vi "findmovablepath.vi"(8 "x":dbl) -> (0 "shift":dbl, 3 "theta handle":dbl=0.15)   [LabVIEW 2012]
uses:
  G_NAV.vi
  G_VEH.vi
  G_PATH.vi
  <vilib>/Analysis/Matrix/Numeric/Conversions/Array To Matrix - RA2.vi
  <vilib>/Analysis/7linalg.llb/Real SVD Decomposition.vi
  G_SEN.vi
  <vilib>/Analysis/NI_AALPro.lvlib
  <vilib>/Analysis/Matrix/NI_Matrix.lvlib
panel:
  out "M6006":T1={"GPSTime"=22892800.0, "attitude[2]"=-0.6123908, "lcc[0]"=-970.47205, "lcc[1]"=200.52362, "heading_GPS"=-0.6106907} {"GPSTime" format="%#_6f"}
  in  "Numeric":dbl
  out "sensor_obs":dbl[][](array[numeric])=[[-2.6493086559458767, 9.313377271515247, 0.316177936945349, -1.2], [-2.6066100840450477, 9.354542103994737, 0.3157590885476819, -1.2], [-2.579340659822815, 9.43207739327695, 0.31450254335468053, -1.2], [-2.6132527619437576, 9.439068677849818, 0.5859163050429868, 1.2000000000000006], [-2.6655003955140795, 9.41719146151926, 0.4953083793337705, 0.40000000000000013], [-2.8189313467074544, 9.344249551531279, 0.5859163050429868, 1.2000000000000006], [-2.5692189092921667, 9.480018973387281, 0.5863351534406539, 1.2000000000000006], [-2.6731933264342116, 9.434269134901442, 0.5863351534406539, 1.2000000000000006], [-2.77635346299322, 9.386711660550553, 0.5863351534406539, 1.2000000000000006], [-2.7290628288714722, 9.419794899689457, 0.5865445776394874, 1.2000000000000006], [-3.035140869949269, 9.26885391372332, 0.5865445776394874, 1.2000000000000006], [-2.550914688564252, 9.509578404068655, 0.3132459981616791, -1.2], [-2.785425991035746, 9.405948172518677, 0.495587629745689, 0.40000000000000013], [-2.7463409502228373, 9.457274042188466, 0.4957970675546278, 0.40000000000000013], [-2.90576588154835, 9.392310316924437, 0.49586688015760744, 0.40000000000000013], [-2.494747129058042, 9.597974241579312, 0.5880105470313224, 1.2000000000000006], [-2.836998990617639, 9.447892074399023, 0.4039934946364334, -0.3999999999999999], [-3.1184925197733824, 9.303796817000539, 0.5880105470313224, 1.2000000000000006], [-2.970577318209098, 9.393517402151646, 0.4960763179665463, 0.40000000000000013], [-2.9699981982750367, 9.392368449256733, 0.588219971230156, 1.2000000000000006], [-3.0729809459427746, 9.340776068194645, 0.4960763179665463, 0.40000000000000013], [-3.1996655181339673, 9.27234939560896, 0.40392368203345375, -0.3999999999999999], [-3.4973819131319495, 9.096981036828707, 0.40392368203345375, -0.3999999999999999], [-2.5289827185611418, 9.605504378157487, 0.3115706045710105, -1.2], [-3.453631348161608, 9.135814142218397, 0.4038538694304742, -0.3999999999999999], [-3.2339632015510937, 9.274656811335685, 0.5886388196278232, 1.2000000000000006], [-2.483097010676977, 9.64588076688389, 0.3111517561733434, -1.2], [-2.8803018639560647, 9.47148380231442, 0.4962857557754851, 0.40000000000000013], [-2.9317308980723027, 9.444962161904348, 0.5888482438266567, 1.2000000000000006], [-2.9582194094409178, 9.433270224287725, 0.4037142442245149, -0.3999999999999999], [-3.0350382771601945, 9.392890956174119, 0.5888482438266567, 1.2000000000000006], [-2.4599617564514022, 9.665942841266034, 0.5890576680254903, 1.2000000000000006], [-3.1930649800894275, 9.320188914278454, 0.5890576680254903, 1.2000000000000006], [-3.424919733239901, 9.200023640728578, 0.4035746190185557, -0.3999999999999999], [-3.4490855593711203, 9.183917089574846, 0.5892670922243238, 1.2000000000000006], [-2.6822275888719656, 9.595825896338217, 0.49649519358442396, 0.40000000000000013], [-3.1777999006997932, 9.352779338748892, 0.40350480641557607, -0.3999999999999999], [-3.3543988506422, 9.251882705008573, 0.5894765164231575, 1.2000000000000006], [-2.4169315260491846, 9.715129108585124, 0.589685940621991, 1.2000000000000006], [-2.4440270491484113, 9.70452412526726, 0.3103140593780091, -1.2], [-2.4445036099706936, 9.705733945395902, 0.40343499381259645, -0.3999999999999999], [-2.8187951120879293, 9.544925625371082, 0.40343499381259645, -0.3999999999999999], [-2.923864294836344, 9.494810195959495, 0.40343499381259645, -0.3999999999999999], [-3.4095769435307015, 9.230983589588824, 0.589685940621991, 1.2000000000000006], [-3.032582634559555, 9.45177853739907, 0.40336518120961684, -0.3999999999999999], [-3.2893092213922506, 9.313834366383366, 0.40336518120961684, -0.3999999999999999], [-3.313999270308597, 9.298296139668594, 0.5898953648208245, 1.2000000000000006], [-2.424651387634039, 9.734980699717582, 0.4967046313933628, 0.40000000000000013], [-2.533097518783729, 9.691715080471495, 0.4967046313933628, 0.40000000000000013], [-2.6407720438905313, 9.646563404831404, 0.4967046313933628, 0.40000000000000013], [-3.4004241638790518, 9.27277469308272, 0.4032255560036576, -0.3999999999999999], [-2.6217419806033297, 9.676437047583807, 0.403155743400678, -0.3999999999999999], [-2.6755410498513874, 9.653323143325384, 0.403155743400678, -0.3999999999999999], [-2.782523848427478, 9.605691332564723, 0.403155743400678, -0.3999999999999999], [-3.072259099823128, 9.465159649093863, 0.496844256599322, 0.40000000000000013], [-3.1500774192579093, 9.424433970288224, 0.403155743400678, -0.3999999999999999], [-3.605192513867668, 9.159018691750026, 0.403155743400678, -0.3999999999999999], [-2.5981277248582337, 9.69583138333276, 0.5907330616161588, 1.2000000000000006], [-3.102875064220138, 9.460567540591395, 0.4030859307976984, -0.3999999999999999], [-3.3599181191701257, 9.319548891673922, 0.4030859307976984, -0.3999999999999999], [-3.385278626883318, 9.304833131837459, 0.49691406920230163, 0.40000000000000013], [-2.5247869108477885, 9.749066890716904, 0.40294630559173916, -0.3999999999999999], [-2.5792234787521573, 9.726796302794572, 0.40294630559173916, -0.3999999999999999], [-3.551164984637863, 9.238618668727831, 0.5913613342126596, 1.2000000000000006], [-2.394482152160173, 9.820127604989409, 0.5915707584114931, 1.2000000000000006], [-2.7494727028492556, 9.675416799445248, 0.40280668038577994, -0.3999999999999999], [-3.681670154810481, 9.169274879714472, 0.40280668038577994, -0.3999999999999999], [-2.349619394154346, 9.868922054648976, 0.5921990310079939, 1.2000000000000006], [-2.625703441413957, 9.761592003343525, 0.497402757423159, 0.40000000000000013], [-3.2137622211581482, 9.48110235361721, 0.497402757423159, 0.40000000000000013], [-3.7275762623275384, 9.185498662423365, 0.5924084552068274, 1.2000000000000006], [-2.3569997188774257, 9.88892730018629, 0.4975423826291182, 0.40000000000000013], [-3.6331178758069624, 9.258143332791025, 0.5926178794056609, 1.2000000000000006], [-3.280263464375405, 9.479130763175284, 0.4976121952320978, 0.40000000000000013], [-2.450699178158054, 9.884289629873633, 0.30675384799783845, -1.2], [-2.4511770399787394, 9.885534502477135, 0.40224817956194303, -0.3999999999999999], [-2.5345511058394776, 9.852902522117958, 0.49775182043805705, 0.40000000000000013], [-3.824786250125524, 9.17047880734031, 0.40224817956194303, -0.3999999999999999], [-2.405397050205525, 9.933526651907876, 0.3061255754013377, -1.2], [-3.4089243051435196, 9.464380504252652, 0.4979612582469959, 0.40000000000000013], [-3.56907303823246, 9.381650335067114, 0.4980310708499755, 0.40000000000000013], [-3.532949127216187, 9.438353586460368, 0.49824050865891434, 0.40000000000000013], [-3.737313762681747, 9.3103050041449, 0.5947121213939967, 1.2000000000000006], [-2.2908474536598415, 10.059979664182297, 0.595549818189331, 1.2000000000000006], [-2.3765186719612967, 10.02943138812595, 0.3044501818106692, -1.2], [-2.462262709016492, 9.999031326649108, 0.4985197590708328, 0.40000000000000013], [-3.657097646318684, 9.409803942456133, 0.4985197590708328, 0.40000000000000013], [-3.835868568229564, 9.295365230962426, 0.40148024092916723, -0.3999999999999999], [-2.3581413988349413, 10.067967806625958, 0.5961780907858316, 1.2000000000000006], [-3.877029743260587, 9.302385055789298, 0.5961780907858316, 1.2000000000000006], [-3.9331436519651666, 9.276595165706414, 0.5963875149846652, 1.2000000000000006], [-3.425151432335213, 9.616047962173518, 0.4989386346887105, 0.40000000000000013], [-2.3143719287589564, 10.127343415537375, 0.49900844729169014, 0.40000000000000013], [-3.7975482431761254, 9.403949992407117, 0.49900844729169014, 0.40000000000000013], [-3.854407472044735, 9.378948406292697, 0.49907825989466975, 0.40000000000000013], [-2.407763132093687, 10.115274836822742, 0.4008519275023507, -0.3999999999999999], [-2.468901871015975, 10.10337801061548, 0.4007821148993711, -0.3999999999999999], [-2.3890129763037065, 10.15395227178771, 0.4993575103065882, 0.40000000000000013], [-3.777898705712374, 9.487607060347795, 0.4994273229095678, 0.40000000000000013], [-4.0346920104398265, 9.315984499311078, 0.5982723327741674, 1.2000000000000006], [-4.015722357091047, 9.342912286209264, 0.40050286448745265, -0.3999999999999999], [-2.372846250599384, 10.200711102617147, 0.30109939462933205, -1.2], [-2.3833228936159903, 10.23029622982958, 0.4001538014725545, -0.3999999999999999], [-3.9666747963375277, 9.4365483588187, 0.4998461985274455, 0.40000000000000013], [-2.30100181314674, 10.278532756817912, 0.5999477263648358, 1.2000000000000006], [-4.109576508398126, 9.423930057048132, 0.5003348867483028, 0.40000000000000013], [-2.35334151682133, 10.334600032038626, 0.2985863042433292, -1.2], [-4.074608378760497, 9.48436394539886, 0.5005443245572416, 0.40000000000000013], [-2.3368079650044735, 10.384014278769136, 0.5007537623661805, 0.40000000000000013], [-2.370078405901655, 10.38320748736416, 0.39917642503083994, -0.3999999999999999], [-4.204212822255533, 9.504238162023881, 0.3988273620159418, -0.3999999999999999], [-2.2707767805352264, 10.48873231405309, 0.2960732138573263, -1.2], [-2.3200348724405737, 10.53572713543776, 0.6051833313356751, 1.2000000000000006], [-2.245779677656643, 10.622703152908741, 0.29356012347132354, -1.2], [-2.279884830624796, 10.622358187824348, 0.6066493007275101, 1.2000000000000006], [-2.358065997017253, 10.651060149761754, 0.5025688900436505, 0.40000000000000013], [-2.206922249961846, 10.718517420078616, 0.29188472988065495, -1.2], [-2.310815072326706, 10.718984235455277, 0.5029179530585486, 0.40000000000000013], [-2.250256927274077, 10.7470116403635, 0.6089529669146794, 1.2000000000000006], [-2.4078141528407944, 10.696197951674801, 0.2910470330853207, -1.2], [-2.2625570787999116, 10.786624601979373, 0.5032670160734467, 0.40000000000000013], [-2.37319268235858, 10.803936049039782, 0.3963839209116553, -0.3999999999999999], [-2.4400133449020482, 10.792431192800741, 0.3963141083086757, -0.3999999999999999], [-2.3484550625403937, 10.948347869936686, 0.3954763570729203, -0.3999999999999999], [-2.2532005442925973, 10.986565753726355, 0.6137697234878515, 1.2000000000000006], [-2.2241527610867795, 11.130722431723722, 0.6164922380726879, 1.2000000000000006], [-2.3272220554510197, 11.112000353866012, 0.3944291680282261, -0.3999999999999999], [-2.2968682826047866, 11.131657762965752, 0.5056406445747536, 0.40000000000000013], [-2.2805508875817773, 11.32421563798276, 0.5068972714283867, 0.40000000000000013], [-2.3203488195890745, 11.3333663356091, 0.39296310336565415, -0.3999999999999999], [-2.2253235316083524, 11.390402063747686, 0.6217278430435271, 1.2000000000000006], [-2.23390046248441, 11.420813566670208, 0.5074557722522236, 0.40000000000000013], [-2.315297365324197, 11.574401473618405, 0.391357413497123, -0.3999999999999999], [-2.2168668356954866, 11.63137340411444, 0.6265445996166993, 1.2000000000000006], [-2.3994033185138965, 11.600249851280598, 0.2730365519856337, -1.2], [-2.233080590823236, 11.690844769333019, 0.5092708999296937, 0.40000000000000013], [-2.3589382981537037, 11.726595493110718, 0.27073288579846444, -1.2], [-2.3008663461775223, 11.796656013544418, 0.38989134883455107, -0.3999999999999999], [-2.209460232985442, 11.892117815907735, 0.6317802045875385, 1.2000000000000006], [-2.2516708194251622, 11.903349900014954, 0.3892630354077345, -0.3999999999999999], [-2.324463966690179, 11.881746284197003, 0.26780094701479445, -1.2], [-2.2175289279374653, 11.922764866099948, 0.5108067771952451, 0.40000000000000013], [-2.2538194745555633, 11.911368790129554, 0.2675915228159609, -1.2], [-2.178403555854863, 12.077484518563601, 0.5117841536369597, 0.40000000000000013], [-2.1829008579162608, 12.095192687788384, 0.6357592643653763, 1.2000000000000006], [-2.2383426880850124, 12.155028982889158, 0.3875875329362237, -0.3999999999999999], [-2.2804615843118747, 12.317890670472249, 0.25921455486261813, -1.2], [-2.2227746224162255, 12.415062075134333, 0.2575391612719496, -1.2], [-2.186230627716147, 12.434387153701119, 0.6426702629268841, 1.2000000000000006], [-2.196164124819029, 12.474982005763925, 0.5145068451531648, 0.40000000000000013], [-2.1425536546232067, 12.599100045840768, 0.6458116259093877, 1.2000000000000006], [-2.2643337612516414, 12.581746676789589, 0.3846554036110799, -0.3999999999999999], [-2.198573038349574, 12.65771577116447, 0.2527224046987775, -1.2], [-2.1750587039156537, 12.73714405461915, 0.5162521602276552, 0.40000000000000013], [-2.238686482838199, 12.824800292270476, 0.38304971374254876, -0.3999999999999999], [-2.1747996213790666, 12.920092091405744, 0.24748679972793824, -1.2], [-2.1535345564869504, 13.01725329936264, 0.6543980180615641, 1.2000000000000006], [-2.187058282696622, 13.165406851352257, 0.519184289552799, 0.40000000000000013], [-2.0682676188644926, 13.230434114169201, 0.24162292216059827, -1.2], [-2.249455724453499, 13.24346320074072, 0.3801873970203845, -0.3999999999999999], [-2.168249294443763, 13.280340530506738, 0.2401569527687633, -1.2], [-2.1361605605328022, 13.338559010168616, 0.6608901682254047, 1.2000000000000006], [-2.1577943406236098, 13.438198159944571, 0.520999417230269, 0.40000000000000013], [-2.1011219599138715, 13.601533356858653, 0.6661257731962439, 1.2000000000000006], [-2.2400954133839512, 13.604417430165359, 0.377743955916098, -0.3999999999999999], [-2.1622288912277443, 13.672487145254262, 0.3773948929011999, -0.3999999999999999], [-2.0809447496291567, 13.728170217410458, 0.23136113641775338, -1.2], [-2.148368119037393, 13.828678025980699, 0.5236522961434944, 0.40000000000000013], [-2.1431530665836362, 14.033933863880375, 0.37495145179691336, -0.3999999999999999], [-2.106513383233814, 14.090157922222986, 0.6761781347402553, 1.2000000000000006], [-2.116678410658171, 14.141260966031997, 0.5257466742328829, 0.40000000000000013], [-2.0736923856429295, 14.42245242291376, 0.6828797091029295, 1.2000000000000006], [-2.0946138788714483, 14.532649102029193, 0.5283995531461083, 0.40000000000000013], [-2.152273017194013, 14.572484794069997, 0.3712513838389937, -0.3999999999999999], [-2.0231688076393577, 14.688270075344283, 0.5293769295878229, 0.40000000000000013], [-2.0756120529212976, 14.699000478760663, 0.37048344520621795, -0.3999999999999999], [-2.0476810196035475, 14.823824383301131, 0.6910472528574387, 1.2000000000000006], [8.784462172926562, 11.47924364037722, 0.6985865240154472, 1.2000000000000006], [8.643867253715156, 11.631338367097312, 0.6985865240154472, 1.2000000000000006], [-2.01182307782236, 15.20812065601524, 0.5329373723397832, 0.40000000000000013], [8.86867671544905, 11.41559660678595, 0.6990053724131143, 1.2000000000000006], [8.58702381954077, 11.72028699299172, 0.6990053724131143, 1.2000000000000006], [8.952448256526495, 11.35108640713428, 0.6994242208107815, 1.2000000000000006], [8.751204607664915, 11.589530329880938, 0.699633645009615, 1.2000000000000006], [-2.0698358361213067, 15.238622346987988, 0.36678337724829835, -0.3999999999999999], [8.78228318958885, 11.618259075505645, 0.5334958731636202, 0.40000000000000013], [9.066064089233228, 11.311820599800757, 0.7006807660037829, 1.2000000000000006], [8.586576710391817, 11.864672700124274, 0.7010996144014501, 1.2000000000000006], [8.904607069385332, 11.588375580628155, 0.5339845613844775, 0.40000000000000013], [8.9823118978036, 11.517019884769494, 0.5340543739874571, 0.40000000000000013], [-2.038520846959818, 15.363492520347437, 0.7021467353956179, 1.2000000000000006], [8.791223365347536, 11.769957155305526, 0.5342638117963959, 0.40000000000000013], [8.577157812432615, 12.002632694506751, 0.7029844321909522, 1.2000000000000006], [9.089521761789143, 11.471296644949536, 0.5344034370023552, 0.40000000000000013], [8.747614402156172, 11.874019031613333, 0.5345430622083145, 0.40000000000000013], [9.196614789945517, 11.42431028033962, 0.5347525000172533, 0.40000000000000013], [8.702856524966558, 11.977947480441758, 0.5348223126202329, 0.40000000000000013], [8.551902917074258, 12.126859885849031, 0.7044504015827872, 1.2000000000000006], [9.301763328727434, 11.37452391977877, 0.7052880983781215, 1.2000000000000006], [8.546058430068586, 12.272774370500398, 0.7065446435711229, 1.2000000000000006], [8.713762205484503, 12.13805016075561, 0.5356600638559883, 0.40000000000000013], [9.379898466547676, 11.440670196564861, 0.5357996890619475, 0.40000000000000013], [8.680290014842434, 12.256372289618902, 0.536078939473866, 0.40000000000000013], [-1.9947666269032363, 15.748326418663561, 0.5366374402977029, 0.40000000000000013], [5.4033137061696035, 14.702228724352713, 0.7105237033489606, 1.2000000000000006], [5.31065139179097, 14.760192151279867, 0.5369166907096213, 0.40000000000000013], [5.318145573506214, 14.776082090179019, 0.7111519759454614, 1.2000000000000006], [5.372647557345696, 14.763989846509837, 0.36287387148143985, -0.3999999999999999], [5.430433378499369, 14.758453624273042, 0.5372657537245195, 0.40000000000000013], [5.282599535397169, 14.828571261939807, 0.3627342462754806, -0.3999999999999999], [-2.0630447970868317, 15.828269580660534, 0.3627342462754806, -0.3999999999999999], [-2.0425899368277762, 16.04197255374355, 0.7161781567174671, 1.2000000000000006], [8.986023479525567, 16.697743175440838, 0.7844504455372108, 1.2000000000000006], [8.870510744967275, 16.775657498704163, 0.7844504455372108, 1.2000000000000006], [8.776249405862337, 16.886004939029128, 0.7852881423325451, 1.2000000000000006], [9.255378545456706, 16.596057732863006, 0.7859164149290457, 1.2000000000000006], [9.146441633836046, 16.684541131912827, 0.7861258391278794, 1.2000000000000006], [9.094705994581439, 16.85736482840408, 0.5628171664150587, 0.40000000000000013], [9.445245140600367, 16.620273164434607, 0.7886389295138823, 1.2000000000000006], [8.745638718171325, 17.096618222434593, 0.7886389295138823, 1.2000000000000006], [9.250822015437112, 16.835004830220694, 0.563305854635916, 0.40000000000000013], [8.898582257650931, 17.072593546817984, 0.563305854635916, 0.40000000000000013], [9.372609476756939, 16.761935663932476, 0.5633756672388956, 0.40000000000000013], [9.022240713238299, 17.00273744358763, 0.5633756672388956, 0.40000000000000013], [9.671704217358442, 16.690540187776413, 0.79261798929172, 1.2000000000000006], [8.733353836557999, 17.341528099528503, 0.7928274134905535, 1.2000000000000006], [9.575618663038583, 16.801373411419853, 0.5644228562835899, 0.40000000000000013], [8.86635551362631, 17.284293500790973, 0.5644228562835899, 0.40000000000000013], [-11.730647795102412, 15.437193920648374, 0.09942389115260453, -1.2], [-11.753961919567294, 15.46091854606451, 0.3329242648031848, -0.3999999999999999], [-2.6376199176507695, 22.880864643377365, 0.586553451428128, 0.40000000000000013], [-2.8095170709695823, 22.87690194098971, 0.5866930766340872, 0.40000000000000013], [-2.472177558679492, 22.932903386537202, 0.5867628892370669, 0.40000000000000013], [-2.1457138125258957, 23.092372962417727, 0.5876006404728222, 0.40000000000000013], [-1.975660428365826, 23.120301035359756, 0.5876704530758019, 0.40000000000000013], [-2.830488522803034, 23.021539526550544, 0.8631939442986329, 1.2000000000000006], [-2.321307029798844, 23.112624067398425, 0.5878798908847407, 0.40000000000000013], [-2.664069979468923, 23.075216022238337, 0.8638222168951337, 1.2000000000000006], [-2.4981915740055283, 23.137390254704062, 0.864659913690468, 1.2000000000000006], [-2.3314305321547493, 23.198157106933053, 0.8654976104858023, 1.2000000000000006], [-1.8217528316749911, 23.325992950774253, 0.5889968925324145, 0.40000000000000013], [-2.1768599709453524, 23.37676650480826, 0.8688483976671393, 1.2000000000000006], [-15.001217509405912, 16.7719561296704, 0.31016535623183017, -0.3999999999999999], [-15.131558329077535, 16.65366297795977, 0.31002573102587094, -0.3999999999999999], [-14.921984448489132, 16.935815146369087, 0.30981629321693205, -0.3999999999999999], [-15.241790010790758, 16.749485916960253, 0.026963118356189475, -1.2], [-15.133075455565274, 16.88861418597005, 0.0267536941573559, -1.2], [-15.017973364486107, 17.261437164441947, 0.3077917277305232, -0.3999999999999999], [9.64601974480163, 21.452115753566822, 0.5922780848724565, 0.40000000000000013], [9.496453028675626, 21.54978831901161, 0.8772253656204823, 1.2000000000000006], [9.33857931433906, 21.631972172843444, 0.8772253656204823, 1.2000000000000006], [9.17999443103193, 21.712775206793534, 0.8772253656204823, 1.2000000000000006], [-15.156829567346312, 17.1472706411717, 0.022774634379518044, -1.2], [9.377029264437805, 21.70662736414938, 0.5929762109022526, 0.40000000000000013], [9.544865059367709, 21.641804454240944, 0.5931158361082118, 0.40000000000000013], [9.710389454590258, 21.571913609233842, 0.8797384560064849, 1.2000000000000006], [-1.8772014233671248, 23.929435618135358, 0.8797384560064849, 1.2000000000000006], [9.095883042737146, 21.944626194626313, 0.8807855770006529, 1.2000000000000006], [9.271801932592034, 21.894917952170292, 0.5938139621380081, 0.40000000000000013], [-15.236180272734178, 17.461386956855613, 0.017120181011011648, -1.2], [9.194957789557106, 22.145529906980062, 0.5951404015946207, 0.40000000000000013], [5.3379716006680615, 24.14040468850077, 0.30115953044745974, -0.3999999999999999], [5.346343602955266, 24.94301298686431, 0.29571414741504976, -0.3999999999999999], [-16.03827076279453, 20.400810973707614, 0.28733663505749585, -0.3999999999999999], [-15.917453817284267, 20.56937941691859, 0.2870573846455774, -0.3999999999999999], [-15.794914133758107, 20.737124067829413, 0.28677813423365894, -0.3999999999999999], [-14.857892347507073, 21.847969012040384, 0.2851724443651278, -0.3999999999999999], [-15.023801434595246, 21.725328510394597, 0.2851026317621482, -0.3999999999999999], [-15.339589077483758, 21.460351215716504, 0.2851026317621482, -0.3999999999999999], [-15.650704132941332, 21.189903024072276, 0.2851026317621482, -0.3999999999999999], [-15.201556508849778, 21.61650958244562, 0.28489319395320933, -0.3999999999999999], [-14.728337374906722, 22.016057756865447, 0.2848233813502297, -0.3999999999999999], [-15.626945243640977, 21.4767441096572, 0.28370637970255586, -0.3999999999999999], [9.50763508171292, 26.73975570562619, 0.6252994460818146, 0.40000000000000013], [-1.4252219468434035, 28.59895493907886, 0.6255088838907534, 0.40000000000000013], [9.725543674751258, 26.692789231824694, 0.6255786964937331, 0.40000000000000013], [9.943355423856874, 26.64378657215293, 0.6258579469056516, 0.40000000000000013], [9.334114379546264, 26.89614247546073, 0.6258579469056516, 0.40000000000000013], [9.216574706656742, 27.200382540182076, 0.6275334493771623, 0.40000000000000013], [10.040081267648652, 26.868922071117122, 0.9827751618326013, 1.2000000000000006], [-1.4946609322957394, 29.821814277404098, 1.0022516123241232, 1.2000000000000006], [9.883884675811041, 31.803099088007194, 0.6592981837328874, 0.40000000000000013], [9.665449175747526, 31.97349509801759, 0.659926497159704, 0.40000000000000013], [10.174424429491456, 31.838119222564067, 0.6602057475716224, 0.40000000000000013], [10.17244090528941, 31.83259465007272, 1.0805762626878783, 1.2000000000000006], [-1.0364518801246452, 37.42334336490329, 0.6869439745128152, 0.40000000000000013], [10.026103833352638, 36.8130958059697, 0.6928780457660825, 0.40000000000000013], [9.743408822772697, 36.92812129013003, 0.6930874835750214, 0.40000000000000013], [10.347031193921643, 36.82288619877287, 1.1808904539291583, 1.2000000000000006], [-21.069030510629236, 31.45954783569295, 0.20558607696836614, -0.3999999999999999], [-21.391355310423045, 31.377757000004777, 0.20467851312963112, -0.3999999999999999], [10.4210427571751, 41.72394225688742, 0.7265975330052368, 0.40000000000000013], [10.107451026305094, 41.89078819565647, 0.7271560338290737, 0.40000000000000013], [10.474235594988285, 41.919051326913184, 1.284136583954108, 1.2000000000000006], [10.13857155297352, 42.00899223589921, 1.284136583954108, 1.2000000000000006], [10.830210018606069, 41.90102810572798, 0.7285522858886659, 0.40000000000000013], [-0.709038750028526, 57.66347671663537, 1.5846603092802805, 1.2000000000000006], [11.120605021860856, 56.96437033164037, 0.8312466248716806, 0.40000000000000013], [-0.7151980727209852, 58.133987434462625, 0.8314560626806193, 0.40000000000000013], [1.5195348183779678, 61.52869356204023, 0.04473783970333195, -0.3999999999999999], [5.073212151726797, 61.48708023724171, 0.04362083805565814, -0.3999999999999999], [11.439817695944253, 61.011847285540675, 0.8593811038724656, 0.40000000000000013], [11.689176472740309, 65.06866600393317, 0.8875155828732506, 0.40000000000000013], [14.49832831315618, 65.07219891982305, 1.7750269060199955, 1.2000000000000006], [8.818111571073048, 72.81602044955893, 1.9136657256478184, 1.2000000000000006], [12.551831810983316, 72.91253923612891, 0.9424581014182081, 0.40000000000000013], [13.768405529858791, 72.71844886386302, 1.9283254195661683, 1.2000000000000006], [1.2476421313017925, 74.97736983119862, -0.04909029870127124, -0.3999999999999999], [0.9387629168292289, 75.21210795753403, 0.9506959885698028, 0.40000000000000013], [17.77975821366545, 76.1598746565128, 2.0169118556727685, 1.2000000000000006], [47.35648972259149, 63.571420836353425, 2.052304545275642, 1.2000000000000006], [13.031972557350265, 79.3416128979354, 2.061938058421986, 1.2000000000000006], [24.83184721270082, 81.07466865802802, 2.156178947897092, 1.2000000000000006], [13.551875448365177, 86.71163580640813, 1.0385900557211387, 0.40000000000000013], [52.872675769586, 69.37798867554798, 2.2194250559448303, 1.2000000000000006], [8.915518332671137, 92.0400907270114, 1.0712623539155988, 0.40000000000000013], [9.692181670683942, 91.99867908899289, 1.0715416043275172, 0.40000000000000013], [20.71894414488982, 95.06455786989261, 2.4164932270472192, 1.2000000000000006], [19.150342204408794, 95.56882049865551, 2.4198440142285564, 1.2000000000000006], [23.490178905085354, 95.9928006820069, 2.448953977866423, 1.2000000000000006], [26.036285319817722, 95.81770414584793, 2.4592157636092677, 1.2000000000000006], [14.717578948116746, 99.12164584891, 1.1254369338277803, 0.40000000000000013], [20.65463162219833, 155.2673630873944, 3.658378726130288, 1.2000000000000006], [12.312708261276875, 191.3556263648354, 4.393457664036117, 1.2000000000000006], [14.978259637770336, 232.0240814937235, 2.048848233439155, 0.40000000000000013], [33.73593705129936, 288.53349296533526, 2.4538311433239053, 0.40000000000000013], [8.92096999050232, 17.23708913161584, 0.3356469563193898, -0.3999999999999999], [-2.5256202703736608, 22.68399055587274, 0.31491261323444397, -0.3999999999999999], [-1.8996165215080512, 23.228271875851924, 0.3116314208944021, -0.3999999999999999], [-3.0296332585078587, 23.183843349397314, 0.8671730040764709, 1.2000000000000006], [5.104128617356655, 23.236200962780366, 0.022984058578351618, -1.2], [-1.2548826959515347, 24.01715071826592, 0.01942384719818102, -1.2], [5.221948215230284, 24.444090337557157, -0.0021468452816766903, -1.2], [-2.224688830349968, 25.593404278777417, 0.9151311456093583, 1.2000000000000006], [5.209357772395169, 25.198536731676327, -0.017434811796527283, -1.2], [-1.1725915542855405, 25.874379726198075, -0.019319629586029397, -1.2], [-15.005798944565672, 21.383214801932546, -0.039005504276384995, -1.2], [-14.976356804490646, 21.66777357175441, -0.04319398825305637, -1.2], [-14.955664951264778, 21.9687081224078, -0.04780132062739484, -1.2], [9.275033221452706, 26.45651279141699, 0.277143995022472, -0.3999999999999999], [9.363878146139614, 27.271589550954324, 0.2716287993870824, -0.3999999999999999], [9.371321144452127, 28.564736959442584, 0.26318147442654893, -0.3999999999999999], [10.747513637749273, 30.43885569655537, 1.0575396008161857, 1.2000000000000006], [11.012472531760006, 30.418068389611857, 1.0592149944068543, 1.2000000000000006], [11.266285997376329, 30.367042635463775, 1.060262115401022, 1.2000000000000006], [-20.735017036098906, 31.521767273772653, 0.20663326601306034, -0.3999999999999999], [-20.49557227262787, 31.709735125755284, 0.20656345341008076, -0.3999999999999999], [10.724864676049275, 37.00446773130826, 0.6956007372822874, 0.40000000000000013], [-21.806198041420327, 31.41066071306105, 0.20272376024620187, -0.3999999999999999], [10.97816933233072, 46.72664514439962, 0.7613642092890853, 0.40000000000000013], [-33.95444016665767, 37.454440166657676, 0.11475988049188635, -0.3999999999999999], [-33.46782468155926, 38.15694699438283, 0.11364287884421248, -0.3999999999999999], [-32.258000408687934, 39.32613895725404, 0.11343344103527364, -0.3999999999999999], [-34.39923085728631, 37.30403001674005, 0.11329381582931441, -0.3999999999999999], [11.618566184124763, 57.01187131155995, 0.8322938139163747, 0.40000000000000013], [16.615400312068406, 60.50485600252477, 1.6937703168725702, 1.2000000000000006], [13.205163345895427, 64.3192947748755, 1.7536656377389712, 1.2000000000000006], [20.538690765112868, 64.00503191176435, 1.7884300547453438, 1.2000000000000006], [13.026046392769018, 79.30712465157343, 0.9869985421192027, 0.40000000000000013], [27.29899080749756, 81.67230442986731, 2.1844512147396244, 1.2000000000000006], [33.69042505267091, 80.06731529671714, 2.2022522716404778, 1.2000000000000006], [29.157427120978678, 82.5346645544511, 2.2146082993716583, 1.2000000000000006], [27.17382907061827, 93.78874887901951, 2.425079619199396, 1.2000000000000006], [34.761055666251615, 92.88790635480824, 2.4590063394104344, 1.2000000000000006], [-2.729118001525531, 22.918683596868465, 0.31309748555697403, -0.3999999999999999], [9.124522914489708, 21.80096170236561, 0.3072332269066863, -0.3999999999999999], [-1.5170192378515415, 28.303045293335575, 0.2765156815956554, -0.3999999999999999], [-1.3900091234452605, 30.022954081648294, 0.2645777264861412, -0.3999999999999999], [4.034616118215339, 61.19769858054814, 0.04620390436590388, -0.3999999999999999], [26.121526235859253, 82.71602090547535, 2.197226090868472, 1.2000000000000006]]
  out "xplot":cluster{dbl[]}[](array[cluster])
  out "yplot":cluster{dbl[]}[](array[cluster])
  out "thetaseed":dbl[](array[numeric])
  out "center":i16
  out "right":i16
  out "left":i16
  out "XY Graph":cluster{"Y":dbl[], "Y":dbl[]}[](graph)=[{"Y"=[0.0], "Y"=[1000.0]}, {"Y"=[], "Y"=[]}, {"Y"=[], "Y"=[]}, {"Y"=[55.79381017995934], "Y"=[-143.41137512848826]}, {"Y"=[1.8243630881955273], "Y"=[-0.6091599202647308]}, {"Y"=[60.825233010671326, 56.37330625127248, 55.349089235151354, 59.801015994550255, 60.825233010671326], "Y"=[-144.72018116547483, -142.44414335187238, -144.44751039360185, -146.72354820720435, -144.72018116547483]}, {"Y"=[0.0, 2.210107140854234e-06, 8.840428449730098e-06, 1.9890964154001267e-05, 3.536171391260723e-05, 5.5252677611861145e-05, 7.956385525176302e-05, 0.00010829524660493917, 0.00014144685155770276, 0.0001790186695416196, 0.00022101070067037654, 0.00026742294460291305, 0.00031825540077079495, 0.00037350806894664856, 0.0004331809489031002, 0.0004972740399580289, 0.0005657873416566872, 0.0006387208537717015, 0.0007160745756209508, 0.0007978485066360008, 0.0008840426462484174, 0.0009746569938897665, 0.0010696915488779268, 0.0011691463105307776, 0.0012730212781661976, 0.001381316451102066, 0.0014940318285425747, 0.0016111674095782291, 0.0017327231935269083, 0.0018586991794791174, 0.001989095366525362, 0.00212391175364246, 0.002263148340148291, 0.0024068051247922995, 0.002554882106551304, 0.0027073792846294964, 0.002864296657776322, 0.003025634224741225, 0.003191391984614711, 0.0033615699362599116, 0.003536168078198898, 0.0037151864094084885, 0.003898624928524441, 0.004086483634296201, 0.004278762525359525, 0.004475461600350172, 0.0046765808579039, 0.004882120296656467, 0.0050920799150162566, 0.00530645971150534, 0.005525259684645789, 0.005748479832959674, 0.005976120154741693, 0.006208180648513917, 0.006444661312457356, 0.006685562145094082, 0.006930883144491418, 0.007180624309171435, 0.007434785636974084, 0.007693367126535122, 0.007956368775921874, 0.008223790583087975, 0.008495632546100751, 0.008771894663368585, 0.009052576932504053, 0.00933767935191554, 0.009627201919329309, 0.009921144632812684, 0.010219507490205615, 0.010522290489461739, 0.010829493628421005, 0.011141116904923365, 0.011457160316581394, 0.011777623861462416, 0.012102507536951634, 0.012431811341116372, 0.012765535271228146, 0.013103679325240591, 0.0134462435006526, 0.013793227794963059, 0.014144632205784546, 0.014500456730615952, 0.014860701366956164, 0.015225366112190386, 0.015594450963703821, 0.015967955919109045, 0.0163458809754502, 0.016728226130226176, 0.017114991380822175, 0.017506176724168654, 0.0179017821577645, 0.018301807678767545, 0.018706253284335617, 0.019115118971512857, 0.019528404737457095, 0.01994611057932616, 0.02036823649393682, 0.02079478247856059, 0.021225748530014243, 0.02166113464522823, 0.022100940821246695], "Y"=[0.0, 0.05249999993797367, 0.10499999950378934, 0.15749999832528905, 0.2099999960303148, 0.26249999224670867, 0.31499998660231265, 0.3674999787249688, 0.41999996824251923, 0.472499954782806, 0.5249999379736712, 0.577499917442957, 0.6299998928185055, 0.682499863728159, 0.7349998297997596, 0.7874997906611497, 0.8399997459401715, 0.8924996952646672, 0.9449996382624795, 0.9974995745614504, 1.0499995037894228, 1.1024994255742389, 1.1549993395437415, 1.2074992453257731, 1.2599991425481762, 1.3124990308387938, 1.3649989098254687, 1.4174987791360436, 1.4699986383983614, 1.5224984872402658, 1.574998325289599, 1.6274981521742047, 1.6799979675219257, 1.7324977709606055, 1.784997562118088, 1.837497340622216, 1.8899971061008334, 1.9424968581817836, 1.994996596492911, 2.047496320662059, 2.099996030317072, 2.152495725085793, 2.204995404596067, 2.2574950684757384, 2.309994716352652, 2.3624943478546507, 2.414993962609581, 2.467493560245286, 2.519993140389611, 2.5724927026704023, 2.6249922467155042, 2.6774917721527607, 2.7299912786100196, 2.7824907657151243, 2.834990233095921, 2.887489680380256, 2.939989107195975, 2.9924885131709242, 3.0449878979329497, 3.0974872611098974, 3.1499866023296144, 3.2024859212199472, 3.2549852174087435, 3.3074844905238483, 3.3599837401931105, 3.412482966044377, 3.464982167705495, 3.5174813448043127, 3.5699804969686775, 3.6224796238264374, 3.6749787250054404, 3.7274778001335362, 3.7799768488385714, 3.8324758707483966, 3.884974865490859, 3.9374738326938097, 3.989972771985096, 4.042471682992569, 4.094970565344078, 4.147469418667473, 4.199968242590603, 4.2524670367413195, 4.304965800747474, 4.3574645342369145, 4.409963236837495, 4.4624619081770645, 4.514960547883476, 4.567459155584579, 4.6199577309082285, 4.672456273482274, 4.724954782934569, 4.777453258892966, 4.829951700985317, 4.882450108839476, 4.934948482083297, 4.987446820344632, 5.039945123251335, 5.09244339043126, 5.144941621512262, 5.197439816122197, 5.249937973888915]}, {"Y"=[55.85492946607054, 56.300112183962334, 56.74529490185413, 57.19047761974598, 57.635660337637766, 58.08084305552956, 58.52602577342136, 58.97120849131315, 59.416391209205, 59.8615739270968, 60.306756644988596, 60.75193936288038, 61.197122080772175, 61.64230479866403, 62.087487516555825, 62.532670234447615, 62.97785295233941, 63.423035670231265, 63.86821838812306, 64.31340110601485, 64.75858382390665, 65.20376654179844, 65.64894925969023, 66.09413197758208, 66.53931469547388, 66.98449741336567, 67.42968013125746, 67.87486284914931, 68.3200455670411, 68.7652282849329, 69.2104110028247, 69.65559372071655, 70.10077643860835, 70.54595915650015, 70.99114187439193, 71.43632459228371, 71.88150731017556, 72.32669002806736, 72.77187274595916, 73.21705546385095], "Y"=[-143.26925304077835, -143.49687629901547, -143.72449955725253, -143.95212281548962, -144.17974607372668, -144.40736933196374, -144.63499259020085, -144.8626158484379, -145.090239106675, -145.3178623649121, -145.54548562314918, -145.7731088813862, -146.00073213962332, -146.22835539786038, -146.45597865609744, -146.68360191433456, -146.91122517257162, -147.1388484308087, -147.36647168904577, -147.59409494728285, -147.82171820551994, -148.04934146375703, -148.27696472199406, -148.50458798023115, -148.73221123846827, -148.9598344967053, -149.18745775494241, -149.4150810131795, -149.64270427141656, -149.87032752965362, -150.09795078789074, -150.3255740461278, -150.55319730436486, -150.78082056260195, -151.00844382083903, -151.23606707907612, -151.46369033731318, -151.6913135955503, -151.91893685378736, -152.14656011202442]}, {"Y"=[46.95734422441421, 47.0463827596022, 47.13542129479015, 47.224459829978144, 47.31349836516614, 47.40253690035408, 47.49157543554208, 47.58061397073008, 47.669652505918016, 47.75869104110601, 47.84772957629395, 47.936768111481946, 48.02580664666995, 48.11484518185789, 48.20388371704588, 48.292922252233886, 48.381960787421825, 48.47099932260982, 48.56003785779782, 48.64907639298576, 48.73811492817376, 48.827153463361746, 48.91619199854969, 49.00523053373769, 49.09426906892568, 49.18330760411363, 49.272346139301625, 49.361384674489564, 49.45042320967757, 49.53946174486556, 49.6285002800535, 49.717538815241504, 49.8065773504295, 49.89561588561743, 49.984654420805434, 50.07369295599343, 50.16273149118137, 50.251770026369364, 50.34080856155737, 50.429847096745306, 50.5188856319333, 50.607924167121304, 50.69696270230924, 50.78600123749724, 50.875039772685184, 50.96407830787318, 51.05311684306117, 51.142155378249115, 51.23119391343711, 51.320232448625106, 51.40927098381305, 51.49830951900105, 51.58734805418904, 51.67638658937698, 51.765425124564985, 51.85446365975298, 51.94350219494092, 52.03254073012892, 52.12157926531691, 52.21061780050485, 52.29965633569285, 52.38869487088079, 52.477733406068786, 52.56677194125679, 52.65581047644473, 52.74484901163272, 52.833887546820726, 52.922926082008665, 53.01196461719666, 53.10100315238466, 53.190041687572595, 53.27908022276059, 53.36811875794859, 53.45715729313653, 53.54619582832453, 53.635234363512524, 53.72427289870047, 53.813311433888465, 53.902349969076404, 53.99138850426441, 54.0804270394524, 54.16946557464034, 54.25850410982834, 54.34754264501633, 54.43658118020427, 54.525619715392274, 54.61465825058027, 54.70369678576821, 54.792735320956204, 54.88177385614421, 54.970812391332146, 55.05985092652014, 55.148889461708144, 55.23792799689608, 55.32696653208408, 55.41600506727202, 55.50504360246001, 55.59408213764801, 55.683120672835955, 55.77215920802395, 55.861197743211946, 55.95023627839994, 56.03927481358789, 56.12831334877588, 56.21735188396388, 56.306390419151825, 56.39542895433982, 56.48446748952781, 56.573506024715755, 56.66254455990375, 56.75158309509169, 56.84062163027969, 56.92966016546769, 57.01869870065563, 57.10773723584363, 57.196775771031625, 57.285814306219564, 57.37485284140757, 57.46389137659556, 57.552929911783494, 57.64196844697149, 57.73100698215949, 57.82004551734743, 57.90908405253543, 58.08716112291137, 58.176199658099364, 58.26523819328731, 58.354276728475305, 58.4433152636633, 58.53235379885125, 58.62139233403924, 58.71043086922723, 58.79946940441518, 58.88850793960317, 58.97754647479111, 59.06658500997911, 59.15562354516711, 59.24466208035505, 59.333700615543044, 59.42273915073105, 59.511777685918986, 59.60081622110698, 59.689854756294984, 59.778893291482916, 59.86793182667091, 59.956970361858914, 60.04600889704685, 60.13504743223485, 60.31312450261079, 60.402163037798786, 60.491201572986725, 60.58024010817473, 60.66927864336272, 60.75831717855066, 60.84735571373866, 60.93639424892665, 61.02543278411459, 61.114471319302595, 61.203509854490534, 61.29254838967853, 61.38158692486653, 61.47062546005447, 61.55966399524247, 61.64870253043047, 61.73774106561841, 61.826779600806404, 61.91581813599439, 62.00485667118234, 62.093895206370334, 62.18293374155833, 62.271972276746276, 62.36101081193427, 62.45004934712227, 62.53908788231021, 62.62812641749821, 62.71716495268615, 62.80620348787415, 62.895242023062146, 62.984280558250084, 63.07331909343808, 63.162357628626076, 63.251396163814015, 63.34043469900201, 63.42947323419001, 63.51851176937796, 63.60755030456595, 63.69658883975394, 63.78562737494189, 63.87466591012988, 63.96370444531783, 64.05274298050581, 64.14178151569382, 64.23082005088176, 64.31985858606976, 64.40889712125775, 64.4979356564457, 64.58697419163369, 64.76505126200964, 64.85408979719762, 64.94312833238557, 65.03216686757357, 65.12120540276156, 65.2102439379495, 65.29928247313751, 65.38832100832549, 65.47735954351344, 65.56639807870144, 65.65543661388938, 65.74447514907737, 65.83351368426537, 65.92255221945331, 66.0115907546413, 66.10062928982931, 66.18966782501724, 66.27870636020525, 66.36774489539324, 66.45678343058118, 66.54582196576918, 66.63486050095719, 66.72389903614511, 66.81293757133312, 66.9019761065211, 66.99101464170904, 67.08005317689705, 67.16909171208498, 67.25813024727299, 67.34716878246098, 67.43620731764892, 67.52524585283692, 67.61428438802493, 67.70332292321285, 67.79236145840086, 67.88139999358886, 67.97043852877678, 68.05947706396479, 68.14851559915279, 68.23755413434073, 68.32659266952872, 68.41563120471668, 68.50466973990466, 68.59370827509267, 68.6827468102806, 68.7717853454686, 68.8608238806566, 68.94986241584455, 69.03890095103253, 69.12793948622053, 69.21697802140848, 69.30601655659646, 69.39505509178447, 69.48409362697241, 69.5731321621604, 69.6621706973484, 69.75120923253635, 69.84024776772434, 69.92928630291229, 70.01832483810027, 70.10736337328828, 70.19640190847622, 70.2854404436642, 70.37447897885221, 70.46351751404015, 70.55255604922814, 70.64159458441614, 70.7306331196041, 70.81967165479207, 70.90871018998008, 70.99774872516802, 71.08678726035602, 71.17582579554401, 71.26486433073195, 71.35390286591995, 71.44294140110789, 71.5319799362959, 71.62101847148388, 71.71005700667183, 71.79909554185983, 71.88813407704782, 71.97717261223576, 72.06621114742377, 72.15524968261175, 72.2442882177997, 72.3333267529877, 72.42236528817568, 72.51140382336364, 72.60044235855163, 72.68948089373963, 72.77851942892757, 72.86755796411556, 72.9565964993035, 73.04563503449151, 73.13467356967949, 73.22371210486745, 73.31275064005544, 73.40178917524342, 73.49082771043138, 73.57986624561937], "Y"=[-138.89375124553214, -138.93927200180423, -138.98479275807625, -139.0303135143483, -139.07583427062036, -139.12135502689242, -139.16687578316444, -139.21239653943653, -139.25791729570855, -139.30343805198058, -139.34895880825266, -139.3944795645247, -139.44000032079677, -139.4855210770688, -139.53104183334085, -139.5765625896129, -139.62208334588496, -139.667604102157, -139.71312485842907, -139.7586456147011, -139.80416637097318, -139.8496871272452, -139.89520788351723, -139.9407286397893, -139.98624939606134, -140.0317701523334, -140.07729090860545, -140.1228116648775, -140.16833242114956, -140.2138531774216, -140.25937393369364, -140.30489468996572, -140.35041544623775, -140.39593620250977, -140.44145695878186, -140.48697771505388, -140.53249847132597, -140.578019227598, -140.62353998387005, -140.66906074014207, -140.71458149641416, -140.76010225268618, -140.80562300895826, -140.8511437652303, -140.89666452150234, -140.9421852777744, -140.98770603404643, -141.0332267903185, -141.07874754659053, -141.1242683028626, -141.16978905913462, -141.2153098154067, -141.26083057167872, -141.3063513279508, -141.35187208422283, -141.3973928404949, -141.44291359676694, -141.48843435303897, -141.53395510931105, -141.57947586558308, -141.62499662185516, -141.67051737812716, -141.71603813439924, -141.76155889067127, -141.80707964694335, -141.85260040321535, -141.89812115948743, -141.94364191575949, -141.9891626720315, -142.0346834283036, -142.08020418457562, -142.1257249408477, -142.1712456971197, -142.21676645339178, -142.2622872096638, -142.3078079659359, -142.3533287222079, -142.39884947847997, -142.44437023475203, -142.48989099102408, -142.53541174729614, -142.58093250356816, -142.62645325984025, -142.67197401611224, -142.71749477238433, -142.76301552865635, -142.80853628492844, -142.85405704120046, -142.89957779747255, -142.94509855374454, -142.99061931001663, -143.03614006628868, -143.0816608225607, -143.1271815788328, -143.17270233510482, -143.2182230913769, -143.2637438476489, -143.30926460392098, -143.354785360193, -143.4003061164651, -143.4458268727371, -143.4913476290092, -143.5368683852812, -143.58238914155328, -143.62790989782533, -143.67343065409736, -143.71895141036944, -143.76447216664147, -143.80999292291352, -143.85551367918555, -143.90103443545763, -143.94655519172966, -143.99207594800174, -144.03759670427374, -144.08311746054582, -144.12863821681785, -144.1741589730899, -144.21967972936199, -144.265200485634, -144.3107212419061, -144.3562419981781, -144.40176275445017, -144.4472835107222, -144.49280426699428, -144.58384577953836, -144.6293665358104, -144.67488729208247, -144.72040804835453, -144.76592880462653, -144.81144956089864, -144.85697031717064, -144.90249107344272, -144.94801182971474, -144.99353258598683, -145.03905334225882, -145.0845740985309, -145.13009485480293, -145.17561561107502, -145.22113636734704, -145.2666571236191, -145.31217787989118, -145.35769863616318, -145.40321939243526, -145.4487401487073, -145.49426090497937, -145.5397816612514, -145.58530241752348, -145.63082317379548, -145.7218646863396, -145.76738544261164, -145.8129061988837, -145.85842695515572, -145.90394771142783, -145.94946846769983, -145.9949892239719, -146.04050998024394, -146.08603073651602, -146.13155149278802, -146.1770722490601, -146.22259300533213, -146.2681137616042, -146.31363451787624, -146.3591552741483, -146.40467603042035, -146.45019678669237, -146.49571754296446, -146.54123829923648, -146.58675905550857, -146.6322798117806, -146.67780056805265, -146.72332132432467, -146.76884208059676, -146.81436283686878, -146.85988359314084, -146.9054043494129, -146.95092510568492, -146.99644586195703, -147.04196661822903, -147.0874873745011, -147.13300813077313, -147.17852888704522, -147.22404964331722, -147.2695703995893, -147.31509115586132, -147.3606119121334, -147.40613266840543, -147.4516534246775, -147.49717418094954, -147.54269493722157, -147.58821569349365, -147.63373644976568, -147.67925720603776, -147.72477796230976, -147.77029871858184, -147.81581947485387, -147.86134023112595, -147.90686098739798, -147.9979024999421, -148.0434232562141, -148.08894401248617, -148.13446476875822, -148.17998552503028, -148.22550628130233, -148.27102703757438, -148.3165477938464, -148.3620685501185, -148.40758930639052, -148.45311006266255, -148.49863081893463, -148.54415157520666, -148.58967233147874, -148.63519308775076, -148.6807138440228, -148.72623460029487, -148.77175535656693, -148.81727611283895, -148.86279686911104, -148.90831762538306, -148.95383838165512, -148.99935913792717, -149.0448798941992, -149.09040065047128, -149.1359214067433, -149.18144216301536, -149.22696291928742, -149.27248367555944, -149.31800443183153, -149.36352518810358, -149.4090459443756, -149.4545667006477, -149.50008745691972, -149.54560821319174, -149.59112896946382, -149.63664972573585, -149.68217048200793, -149.72769123827996, -149.77321199455199, -149.81873275082407, -149.86425350709612, -149.90977426336815, -149.95529501964023, -150.00081577591226, -150.0463365321843, -150.09185728845637, -150.1373780447284, -150.18289880100048, -150.2284195572725, -150.27394031354456, -150.3194610698166, -150.36498182608864, -150.4105025823607, -150.45602333863278, -150.5015440949048, -150.54706485117688, -150.5925856074489, -150.63810636372094, -150.68362711999302, -150.72914787626505, -150.7746686325371, -150.82018938880915, -150.86571014508118, -150.91123090135326, -150.9567516576253, -151.00227241389734, -151.04779317016943, -151.09331392644145, -151.13883468271348, -151.18435543898556, -151.2298761952576, -151.27539695152967, -151.3209177078017, -151.36643846407375, -151.4119592203458, -151.45747997661783, -151.5030007328899, -151.54852148916194, -151.594042245434, -151.63956300170608, -151.6850837579781, -151.73060451425013, -151.77612527052221, -151.82164602679424, -151.8671667830663, -151.91268753933835, -151.95820829561038, -152.00372905188246, -152.04924980815449, -152.09477056442654, -152.14029132069862, -152.18581207697065, -152.23133283324267, -152.27685358951476, -152.32237434578678, -152.36789510205887, -152.4134158583309, -152.45893661460295, -152.504457370875]}, {"Y"=[], "Y"=[]}, {"Y"=[], "Y"=[]}, {"Y"=[], "Y"=[]}, {"Y"=[-16.5, -15.25, -15.0, -13.5, -13.25, -13.25, -13.25, -13.0, -13.0, -12.75, -12.75, -12.75, -12.75, -12.75, -12.75, -12.75, -12.5, -12.5, -12.5, -12.5, -12.5, -12.5, -12.25, -12.25, -12.25, -12.25, -12.25, -12.25, -12.0, -12.0, -12.0, -11.75, -11.75, -11.75, -11.5, -11.5, -11.5, -11.5, -11.5, -11.25, -10.75, -10.75, -10.5, -10.5, -10.25, -10.25, -10.0, -10.0, -10.0, -10.0, -10.0, -9.75, -9.75, -9.75, -9.75, -9.75, -9.75, -9.75, -9.75, -9.75, -9.75, -9.5, -9.5, -9.5, -9.5, -9.5, -9.5, -9.5, -9.5, -9.5, -9.5, -9.5, -9.5, -9.5, -9.5, -9.5, -9.5, -9.5, -9.5, -9.5, -9.25, -9.25, -9.25, -9.25, -9.25, -9.25, -9.25, -9.25, -9.25, -9.25, -9.25, -9.25, -9.25, -9.25, -9.25, -9.25, -9.25, -9.25, -9.25, -9.25, -9.25, -9.25, -9.0, -9.0, -9.0, -9.0, -9.0, -9.0, -9.0, -9.0, -9.0, -9.0, -9.0, -9.0, -9.0, -9.0, -9.0, -9.0, -9.0, -9.0, -9.0, -9.0, -9.0, -9.0, -9.0, -9.0, -9.0, -9.0, -8.75, -8.75, -8.75, -8.75, -8.75, -8.75, -8.75, -8.75, -8.75, -8.75, -8.75, -8.75, -8.75, -8.75, -8.75, -8.75, -8.75, -8.75, -8.75, -8.75, -8.75, -8.75, -8.75, -8.75, -8.75, -8.75, -8.75, -8.75, -8.75, -8.75, -8.75, -8.75, -8.75, -8.75, -8.75, -8.75, -8.75, -8.5, -8.5, -8.5, -8.5, -8.5, -8.5, -8.5, -8.5, -8.5, -8.5, -8.5, -8.5, -8.5, -8.5, -8.5, -8.5, -8.5, -8.5, -8.5, -8.5, -8.5, -8.5, -8.5, -8.5, -8.5, -8.5, -8.5, -8.5, -8.5, -8.5, -8.5, -8.5, -8.5, -8.5, -8.5, -8.5, -8.25, -8.25, -8.25, -8.25, -8.25, -8.25, -8.25, -8.25, -8.25, -8.25, -8.25, -8.25, -8.25, -8.25, -8.25, -8.25, -8.25, -8.25, -8.25, -8.25, -8.25, -8.25, -8.25, -8.25, -8.25, -8.25, -8.25, -8.25, -8.25, -8.25, -8.25, -8.25, -8.25, -8.0, -8.0, -8.0, -8.0, -8.0, -8.0, -8.0, -8.0, -8.0, -8.0, -8.0, -8.0, -8.0, -8.0, -8.0, -8.0, -8.0, -8.0, -8.0, -8.0, -8.0, -8.0, -8.0, -8.0, -8.0, -7.75, -7.75, -7.75, -7.75, -7.75, -7.75, -7.75, -7.75, -7.75, -7.75, -7.75, -7.75, -7.75, -7.75, -7.75, -7.75, -7.75, -7.75, -7.75, -7.75, -7.75, -7.75, -7.75, -7.75, -7.75, -7.75, -7.5, -7.5, -7.5, -7.5, -7.5, -7.5, -7.5, -7.5, -7.5, -7.5, -7.5, -7.5, -7.5, -7.5, -7.5, -7.5, -7.5, -7.5, -7.5, -7.5, -7.5, -7.5, -7.5, -7.5, -7.5, -7.25, -7.25, -7.25, -7.25, -7.25, -7.25, -7.25, -7.25, -7.25, -7.25, -7.25, -7.25, -7.25, -7.25, -7.25, -7.25, -7.25, -7.25, -7.25, -7.25, -7.25, -7.25, -7.25, -7.0, -7.0, -7.0, -7.0, -7.0, -7.0, -7.0, -7.0, -7.0, -7.0, -7.0, -7.0, -7.0, -7.0, -7.0, -7.0, -7.0, -7.0, -7.0, -6.75, -6.75, -6.75, -6.75, -6.75, -6.75, -6.75, -6.75, -6.75, -6.75, -6.75, -6.75, -6.75, -6.75, -6.75, -6.75, -6.75, -6.75, -6.75, -6.75, -6.75, -6.75, -6.75, -6.5, -6.5, -6.5, -6.5, -6.5, -6.5, -6.5, -6.5, -6.5, -6.5, -6.5, -6.5, -6.5, -6.5, -6.5, -6.5, -6.5, -6.5, -6.5, -6.5, -6.5, -6.5, -6.5, -6.5, -6.5, -6.5, -6.5, -6.5, -6.5, -6.5, -6.25, -6.25, -6.25, -6.25, -6.25, -6.25, -6.25, -6.25, -6.25, -6.25, -6.25, -6.25, -6.25, -6.25, -6.25, -6.25, -6.25, -6.0, -6.0, -6.0, -6.0, -6.0, -6.0, -6.0, -6.0, -6.0, -6.0, -6.0, -5.75, -5.75, -5.75, -5.75, -5.75, -5.75, -5.75, -5.75, -5.75, -5.75, -5.5, -5.25, -5.0, -4.75, -4.5, -4.5, -4.25, -4.25, -4.0, -4.0, -3.75, -3.75, -3.5, -3.5, -3.25, -3.25, -3.25, -3.25, -3.0, -3.0, 2.0, 2.0, 2.0, 2.0, 2.0, 2.0, 2.0, 2.25, 2.25, 2.25, 2.25, 2.25, 2.25, 2.25, 2.25, 2.25, 2.25, 2.25, 2.25, 2.25, 2.25, 2.25, 2.25, 2.25, 2.25, 2.25, 2.25, 2.25, 2.25, 2.5, 2.5, 2.5, 2.5, 2.5, 2.5, 2.5, 2.5, 2.5, 2.5, 2.5, 2.5, 2.5, 2.5, 2.5, 2.5, 2.5, 2.5, 2.5, 2.5, 2.5, 2.5, 2.5, 2.5, 2.5, 2.5, 2.5, 2.5, 2.5, 2.5, 2.5, 2.5, 2.5, 2.5, 2.5, 2.5, 2.5, 2.5, 2.5, 2.5, 2.5, 2.5, 2.75, 2.75, 2.75, 2.75, 2.75, 2.75, 2.75, 2.75, 2.75, 2.75, 2.75, 2.75, 2.75, 2.75, 2.75, 2.75, 2.75, 2.75, 2.75, 2.75, 2.75, 2.75, 2.75, 2.75, 2.75, 2.75, 2.75, 2.75, 2.75, 2.75, 2.75, 2.75, 2.75, 2.75, 2.75, 2.75, 2.75, 2.75, 2.75, 2.75, 2.75, 2.75, 2.75, 2.75, 2.75, 2.75, 2.75, 2.75, 2.75, 2.75, 3.0, 3.0, 3.0, 3.0, 3.0, 3.0, 3.0, 3.0, 3.0, 3.0, 3.0, 3.0, 3.0, 3.0, 3.0, 3.0, 3.0, 3.0, 3.0, 3.0, 3.0, 3.0, 3.0, 3.0, 3.0, 3.0, 3.0, 3.0, 3.0, 3.0, 3.0, 3.0, 3.0, 3.0, 3.0, 3.0, 3.0, 3.0, 3.0, 3.0, 3.0, 3.0, 3.0, 3.0, 3.0, 3.0, 3.0, 3.25, 3.25, 3.25, 3.25, 3.25, 3.25, 3.25, 3.25, 3.25, 3.25, 3.25, 3.25, 3.25, 3.25, 3.25, 3.25, 3.25, 3.25, 3.25, 3.25, 3.25, 3.25, 3.25, 3.25, 3.25, 3.25, 3.25, 3.25, 3.25, 3.25, 3.25, 3.25, 3.25, 3.25, 3.25, 3.25, 3.25, 3.25, 3.25, 3.25, 3.25, 3.25, 3.25, 3.25, 3.25, 3.25, 3.25, 3.25, 3.25, 3.25, 3.25, 3.25, 3.25, 3.5, 3.5, 3.5, 3.5, 3.5, 3.5, 3.5, 3.5, 3.5, 3.5, 3.5, 3.5, 3.5, 3.5, 3.5, 3.5, 3.5, 3.5, 3.5, 3.5, 3.5, 3.5, 3.5, 3.5, 3.5, 3.5, 3.5, 3.5, 3.5, 3.5, 3.5, 3.5, 3.5, 3.5, 3.5, 3.5, 3.5, 3.5, 3.5, 3.5, 3.5, 3.5, 3.5, 3.5, 3.5, 3.5, 3.5, 3.5, 3.5, 3.5, 3.5, 3.5, 3.5, 3.5, 3.5, 3.5, 3.5, 3.75, 3.75, 3.75, 3.75, 3.75, 3.75, 3.75, 3.75, 3.75, 3.75, 3.75, 3.75, 3.75, 3.75, 3.75, 3.75, 3.75, 3.75, 3.75, 3.75, 3.75, 3.75, 3.75, 3.75, 3.75, 3.75, 3.75, 3.75, 3.75, 3.75, 3.75, 3.75, 3.75, 3.75, 3.75, 3.75, 3.75, 4.0, 4.0, 4.0, 4.0, 4.0, 4.0, 4.0, 4.0, 4.0, 4.0, 4.0, 4.0, 4.0, 4.0, 4.0, 4.0, 4.0, 4.0, 4.0, 4.0, 4.0, 4.0, 4.0, 4.0, 4.0, 4.0, 4.0, 4.0, 4.0, 4.0, 4.0, 4.0, 4.0, 4.0, 4.0, 4.0, 4.25, 4.25, 4.25, 4.25, 4.25, 4.25, 4.25, 4.25, 4.25, 4.25, 4.25, 4.25, 4.25, 4.25, 4.25, 4.25, 4.25, 4.25, 4.25, 4.25, 4.25, 4.25, 4.25, 4.25, 4.25, 4.25, 4.25, 4.25, 4.25, 4.25, 4.25, 4.25, 4.25, 4.25, 4.25, 4.25, 4.25, 4.25, 4.25, 4.25, 4.25, 4.25, 4.25, 4.5, 4.5, 4.5, 4.5, 4.5, 4.5, 4.5, 4.5, 4.5, 4.5, 4.5, 4.5, 4.5, 4.5, 4.5, 4.5, 4.5, 4.5, 4.5, 4.5, 4.5, 4.5, 4.5, 4.5, 4.5, 4.5, 4.5, 4.75, 4.75, 4.75, 4.75, 4.75, 4.75, 4.75, 4.75, 4.75, 4.75, 4.75, 4.75, 4.75, 4.75, 4.75, 4.75, 4.75, 4.75, 4.75, 4.75, 4.75, 4.75, 4.75, 4.75, 4.75, 4.75, 4.75, 4.75, 4.75, 5.0, 5.0, 5.0, 5.0, 5.0, 5.0, 5.0, 5.0, 5.0, 5.0, 5.0, 5.0, 5.0, 5.0, 5.0, 5.0, 5.0, 5.0, 5.0, 5.0, 5.0, 5.25, 5.25, 5.25, 5.25, 5.25, 5.25, 5.25, 5.25, 5.25, 5.25, 5.25, 5.25, 5.25, 5.25, 5.5, 5.5, 5.5, 5.5, 5.5, 5.5, 5.5, 5.5, 5.5, 5.5, 5.5, 5.5, 5.75, 5.75, 5.75, 5.75, 5.75, 5.75, 5.75, 5.75, 5.75, 5.75, 5.75, 5.75, 5.75, 5.75, 5.75, 5.75, 5.75, 6.0, 6.0, 6.0, 6.0, 6.0, 6.0, 6.0, 6.0, 6.0, 6.0, 6.0, 6.25, 6.25, 6.25, 6.25, 6.25, 6.25, 6.25, 6.25, 6.5, 6.5, 6.5, 6.5, 6.5, 6.5, 6.5, 6.5, 6.5, 6.75, 6.75, 6.75, 6.75, 7.0, 7.0, 7.0, 7.25, 7.25, 7.25, 7.25, 7.25, 7.25, 7.25, 7.5, 7.5, 8.0, 8.0, 8.0, 8.0, 8.0, 8.25, 8.25, 8.5, 8.5, 8.5, 8.75, 8.75, 8.75, 8.75, 8.75, 9.0, 9.0, 9.0, 9.0, 9.0, 9.0, 9.25, 9.25, 9.25, 9.25, 9.25, 9.25, 9.5, 9.5, 9.5, 9.5, 9.5, 9.5, 9.75, 9.75, 9.75, 10.0, 10.0, 10.0, 10.0, 10.25, 10.25, 10.5, 10.5, 10.5, 10.75, 10.75, 10.75, 10.75, 11.0, 11.0, 11.0, 11.0, 11.0, 11.25, 11.25, 11.25, 11.25, 11.25, 11.25, 11.25, 11.25, 11.25, 11.25, 11.5, 11.5, 11.5, 11.5, 11.5, 11.5, 11.5, 11.5, 11.5, 11.5, 11.5, 11.5, 11.5, 11.5, 11.5, 11.75, 11.75, 11.75, 11.75, 11.75, 11.75, 11.75, 11.75, 11.75, 11.75, 11.75, 11.75, 11.75, 11.75, 11.75, 11.75, 11.75, 11.75, 11.75, 11.75, 12.0, 12.0, 12.0, 12.0, 12.0, 12.0, 12.0, 12.0, 12.0, 12.0, 12.0, 12.0, 12.0, 12.0, 12.0, 12.0, 12.0, 12.0, 12.0, 12.0, 12.0, 12.0, 12.0, 12.0, 12.0, 12.0, 12.0, 12.25, 12.25, 12.25, 12.25, 12.25, 12.25, 12.25, 12.25, 12.25, 12.25, 12.25, 12.25, 12.25, 12.25, 12.25, 12.25, 12.5, 12.5, 12.5, 12.5, 12.5, 12.5, 12.5, 12.5, 12.5, 12.5, 12.5, 12.5, 12.5, 12.75, 12.75, 12.75, 12.75, 12.75, 12.75, 12.75, 12.75, 12.75, 12.75, 13.0, 13.0, 13.0, 13.0, 13.0, 13.0, 13.0, 13.0, 13.0, 13.0, 13.0, 13.0, 13.0, 13.0, 13.0, 13.0, 13.0, 13.0, 13.0, 13.0, 13.0, 13.0, 13.0, 13.25, 13.25, 13.25, 13.25, 13.25, 13.25, 13.25, 13.25, 13.25, 13.25, 13.25, 13.25, 13.25, 13.25, 13.25, 13.25, 13.25, 13.25, 13.25, 13.5, 13.5, 13.5, 13.5, 13.5, 13.5, 13.5, 13.5, 13.5, 13.5, 13.75, 13.75, 13.75, 13.75, 13.75, 13.75, 13.75, 13.75, 13.75, 14.0, 14.0, 14.0, 14.0, 14.5, 14.75, 15.5, 15.75, 16.0, 19.25, 19.25, 19.25, 19.5, 19.5, 19.75, 22.25, 22.25, 22.25, 22.5, 22.5, 22.5, 22.75, 22.75, 22.75, 22.75, 23.0, 23.0, 23.0, 23.25, 23.25, 23.25, 23.5, 23.5, 23.5, 23.5, 23.5, 23.5, 23.75, 23.75, 23.75, 23.75, 23.75, 23.75, 23.75, 23.75, 23.75, 23.75, 23.75, 24.0, 24.0, 24.0, 24.0, 24.0, 24.0, 24.0, 24.25, 24.25, 24.5], "Y"=[46.5, 46.5, 46.5, 2.75, 0.5, 2.75, 17.0, 0.75, 17.25, -6.5, -2.25, -1.75, 0.5, 0.75, 1.0, 3.75, -6.5, 0.75, 4.0, 4.25, 17.25, 21.5, -6.75, -6.5, -1.75, 17.25, 21.5, 22.25, -6.75, 21.75, 22.0, -6.5, 11.25, 22.0, 10.5, 10.75, 11.0, 11.5, 11.75, -6.0, 3.75, 8.25, -1.0, 8.25, -1.25, -1.0, -7.0, -1.25, 2.75, 3.0, 3.5, -10.75, -10.5, -10.0, -9.5, -9.25, -8.25, -6.75, -1.25, 3.0, 3.25, -20.5, -15.5, -15.25, -14.75, -10.5, -10.25, -10.0, -9.75, -9.25, -9.0, -8.75, -8.25, -8.0, -7.75, -7.5, -1.0, 0.5, 1.5, 2.75, -20.25, -18.25, -17.75, -17.5, -17.0, -15.75, -15.5, -10.75, -10.25, -9.5, -9.0, -8.75, -8.25, -8.0, -7.75, 0.75, 1.0, 1.25, 2.25, 3.5, 7.25, 7.5, -19.0, -17.5, -17.25, -10.5, -10.25, -10.0, -9.25, -9.0, -8.75, -8.25, -8.0, -7.25, -7.0, -6.75, -4.75, -4.5, -4.25, 0.75, 1.0, 1.25, 1.75, 2.25, 2.5, 2.75, 3.5, 7.5, -17.5, -12.75, -12.0, -11.75, -10.5, -9.75, -9.5, -9.25, -9.0, -8.75, -8.5, -8.25, -8.0, -7.75, -7.5, -7.0, -6.75, -4.75, -4.5, -3.75, -3.25, -3.0, -1.5, -0.5, -0.25, 0.0, 0.25, 1.75, 2.5, 2.75, 4.25, 4.75, 5.5, 5.75, 6.25, 7.5, 7.75, -13.25, -13.0, -12.75, -12.0, -11.75, -8.25, -8.0, -7.0, -6.75, -5.5, -5.0, -4.75, -4.5, -4.0, -3.75, -3.25, -3.0, -2.75, -2.0, -1.75, -1.5, -1.0, -0.5, -0.25, 0.0, 0.25, 0.5, 0.75, 1.75, 2.0, 4.0, 4.25, 4.75, 5.75, 6.0, 6.25, -17.5, -12.75, -12.0, -11.5, -10.25, -8.25, -8.0, -7.75, -5.5, -4.75, -4.0, -3.75, -3.5, -3.25, -3.0, -2.75, -2.5, -2.25, -2.0, -1.75, -1.5, -0.75, -0.5, -0.25, 0.0, 0.25, 0.5, 2.25, 4.5, 4.75, 5.75, 6.0, 6.25, -13.5, -13.25, -13.0, -7.75, -5.75, -5.5, -5.25, -5.0, -4.75, -4.5, -3.75, -3.5, -3.25, -2.25, -2.0, -1.75, -1.5, -1.25, -0.75, -0.5, -0.25, 0.0, 0.25, 0.5, 0.75, -13.25, -12.5, -6.0, -5.75, -5.25, -5.0, -4.75, -4.5, -4.25, -3.25, -2.5, -2.25, -2.0, -1.75, -1.5, -1.25, -0.75, -0.5, -0.25, 0.0, 0.25, 0.5, 4.0, 4.25, 7.75, 8.0, -14.0, -13.25, -13.0, -8.0, -5.25, -5.0, -4.75, -3.75, -3.0, -2.0, -1.75, -1.5, -1.25, -0.5, -0.25, 0.25, 0.5, 0.75, 1.0, 1.25, 1.5, 2.25, 2.5, 3.75, 9.25, -7.75, -7.25, -7.0, -6.75, -6.5, -6.25, -6.0, -5.75, -5.5, -5.25, -5.0, -3.5, -1.75, -1.5, -1.25, -0.5, -0.25, 1.0, 1.25, 1.75, 2.5, 5.75, 8.5, -9.0, -8.0, -7.75, -7.0, -6.75, -6.5, -5.5, -5.25, -5.0, -2.0, -1.75, 1.25, 1.5, 2.5, 4.0, 4.25, 4.5, 6.0, 8.5, -9.25, -9.0, -7.5, -7.25, -5.75, -5.5, -2.75, -2.5, -1.0, -0.75, -0.5, -0.25, 0.0, 1.0, 1.25, 1.75, 2.75, 3.0, 4.5, 4.75, 5.75, 6.0, 6.25, -20.0, -8.0, -7.5, -7.25, -4.5, -4.25, -3.25, -3.0, -2.75, -2.5, -1.25, -1.0, -0.75, -0.5, 2.25, 2.5, 2.75, 3.0, 3.25, 3.5, 3.75, 4.0, 4.25, 4.5, 4.75, 5.0, 5.25, 5.5, 5.75, 6.0, -20.25, -20.0, -14.0, -13.75, -8.0, -7.75, -7.25, -5.0, -4.75, -4.5, -3.5, -3.25, -3.0, -2.0, -1.75, -1.5, 3.0, -20.0, -14.0, -13.75, -8.0, -7.75, -7.5, -7.25, -5.0, -2.0, -1.75, -1.5, -20.5, -20.25, -14.25, -8.0, -7.75, -7.5, -2.0, -1.75, -1.5, 3.0, 3.0, 3.0, 3.0, 3.0, 3.0, 20.75, 3.0, 20.75, 3.0, 20.75, 3.0, 20.75, 3.0, 20.75, 3.0, 21.0, 22.0, 22.25, 3.0, 22.25, -8.25, -8.0, -7.25, -2.75, -2.5, -2.25, -2.0, -20.5, -14.5, -14.25, -8.5, -8.25, -8.0, -7.75, -7.25, -4.5, -4.0, -3.5, -3.25, -3.0, -2.5, -2.25, -2.0, -1.5, -1.25, -1.0, 4.75, 6.0, 6.25, -20.5, -20.25, -14.25, -8.25, -8.0, -7.75, -5.0, -4.5, -4.25, -4.0, -3.75, -3.5, -3.25, -3.0, -2.75, -2.5, -2.25, -2.0, -1.75, -1.5, -1.25, -1.0, -0.75, 0.75, 1.75, 2.0, 2.25, 2.5, 2.75, 3.0, 3.25, 3.5, 3.75, 4.0, 5.0, 5.25, 5.5, 5.75, 6.25, 6.5, 6.75, 7.0, -20.5, -20.25, -14.25, -8.25, -7.75, -4.75, -4.5, -4.25, -4.0, -3.75, -3.5, -3.25, -3.0, -2.75, -2.5, -2.0, -1.75, -1.5, -1.25, -1.0, -0.75, -0.5, 0.25, 0.5, 0.75, 1.0, 1.25, 1.5, 1.75, 2.0, 2.25, 2.5, 2.75, 3.25, 3.5, 3.75, 4.0, 4.25, 4.5, 4.75, 5.0, 5.25, 5.5, 5.75, 6.0, 6.25, 6.5, 6.75, 7.0, 7.25, -20.25, -7.75, -5.25, -4.5, -4.25, -4.0, -3.75, -3.5, -3.25, -2.75, -2.5, -2.25, -2.0, -1.75, -1.5, -1.25, -1.0, -0.75, -0.5, -0.25, 0.0, 0.25, 0.5, 0.75, 1.0, 1.25, 1.5, 1.75, 2.0, 2.25, 2.5, 2.75, 4.25, 4.5, 4.75, 5.0, 5.25, 5.5, 5.75, 6.0, 6.25, 6.5, 6.75, 7.0, 7.5, 9.5, 10.75, -20.5, -7.5, -6.75, -6.0, -5.75, -5.0, -4.75, -4.5, -4.25, -4.0, -3.25, -3.0, -2.75, -2.5, -2.0, -1.75, -1.5, -1.25, -1.0, -0.75, -0.5, -0.25, 0.0, 0.25, 0.5, 0.75, 1.0, 1.25, 1.5, 1.75, 2.0, 2.25, 2.5, 2.75, 3.0, 4.5, 4.75, 5.0, 5.25, 5.5, 5.75, 6.0, 6.25, 6.5, 6.75, 7.0, 7.25, 9.25, 9.5, 10.75, 11.0, 12.25, 12.75, -7.75, -7.5, -6.75, -6.5, -5.75, -5.5, -5.25, -4.75, -4.25, -4.0, -3.5, -3.0, -2.75, -2.25, -2.0, -1.75, -1.5, -1.25, -1.0, -0.75, -0.5, -0.25, 0.0, 0.25, 0.5, 0.75, 1.0, 1.25, 1.5, 1.75, 2.0, 2.25, 2.5, 2.75, 3.0, 4.75, 5.0, 5.25, 5.5, 5.75, 6.0, 6.5, 6.75, 7.0, 8.75, 9.0, 9.25, 10.25, 10.75, 11.0, 11.25, 12.25, 12.5, 12.75, 13.0, 13.25, 13.75, -8.75, -7.5, -6.5, -6.25, -5.5, -5.0, -4.75, -4.5, -4.25, -4.0, -2.25, -1.75, -1.5, -1.25, -1.0, -0.75, -0.5, -0.25, 0.0, 0.25, 0.5, 1.0, 1.25, 1.5, 1.75, 2.0, 2.25, 2.5, 2.75, 3.0, 3.25, 9.75, 11.0, 11.25, 12.25, 12.5, 13.0, -8.5, -7.5, -6.75, -6.5, -5.5, -5.25, -4.25, -4.0, -3.25, -3.0, -2.75, -2.5, -2.25, -1.75, -1.5, -1.25, -1.0, -0.75, -0.5, -0.25, 0.0, 0.25, 0.5, 0.75, 1.0, 1.25, 1.5, 1.75, 2.0, 2.25, 2.5, 2.75, 3.0, 12.5, 13.0, 13.25, -9.75, -9.5, -9.25, -8.75, -8.5, -8.25, -7.75, -7.5, -7.25, -7.0, -6.75, -6.5, -6.25, -6.0, -5.75, -5.0, -4.25, -3.0, -2.75, -2.5, -2.25, -1.75, -1.5, 0.0, 0.25, 0.5, 0.75, 1.0, 1.25, 1.5, 1.75, 2.0, 2.5, 2.75, 3.0, 3.25, 11.0, 11.25, 11.5, 12.0, 12.25, 12.5, 13.0, -10.0, -9.0, -8.75, -8.5, -8.25, -7.5, -7.25, -6.5, -6.0, -5.75, -4.5, -4.25, -4.0, -3.0, 0.25, 0.5, 0.75, 1.0, 2.5, 2.75, 3.0, 3.5, 11.5, 11.75, 12.0, 12.25, 12.75, -11.25, -10.75, -10.0, -9.5, -9.25, -9.0, -8.75, -8.0, -7.25, -7.0, -6.5, -6.25, -6.0, -5.75, -5.5, -4.75, -4.5, -4.25, -4.0, -3.75, 2.25, 2.5, 2.75, 3.0, 3.5, 6.75, 11.25, 11.5, 12.0, -12.25, -9.0, -8.75, -6.5, -6.25, -6.0, -5.75, -5.5, -5.25, -5.0, -4.75, -4.25, -4.0, -3.75, -3.5, 1.25, 2.5, 2.75, 3.25, 6.75, 12.0, -9.0, -8.75, -8.5, -7.0, -5.75, -5.5, -4.25, -3.5, -3.25, -3.0, -0.75, 2.0, 2.25, 12.0, -10.75, -9.0, -8.25, -3.25, -3.0, 2.0, 2.25, 2.5, 4.25, 5.75, 12.0, 13.0, -9.0, -3.5, 1.0, 1.25, 1.5, 1.75, 2.25, 2.5, 2.75, 3.25, 5.5, 5.75, 8.25, 8.5, 8.75, 9.0, 9.25, -9.0, -8.75, 1.5, 1.75, 3.25, 3.5, 5.5, 5.75, 6.25, 8.25, 9.0, -9.0, -8.75, 1.75, 3.25, 3.75, 5.75, 9.0, 9.5, -17.25, 1.5, 1.75, 3.25, 4.75, 5.5, 6.0, 6.25, 6.75, 4.5, 4.75, 5.5, 6.25, 4.5, 4.75, 5.75, 4.5, 6.25, 8.75, 9.0, 10.25, 10.5, 17.0, 4.0, 17.0, 1.5, 6.75, 10.75, 11.0, 17.5, 0.0, 17.5, 3.25, 17.25, 17.5, 0.25, 3.0, 3.25, 11.25, 11.5, -0.5, 6.75, 11.25, 11.5, 12.25, 35.5, -11.25, 12.0, 12.25, 12.75, 17.0, 35.5, -13.0, -12.25, -10.75, 12.0, 12.25, 17.0, 16.5, 16.75, 28.5, 16.25, 16.5, 28.25, 28.75, 28.0, 28.5, 2.25, 28.0, 28.25, 2.0, 2.5, 3.25, 8.0, 2.75, 3.25, 8.0, 8.25, 15.75, -7.75, -7.5, -5.25, -4.75, -2.25, 5.25, 8.0, 8.25, 15.25, 15.5, -9.25, -7.25, -4.75, -3.5, -3.0, -2.5, 2.5, 4.0, 4.25, 4.5, 4.75, 7.0, 7.75, 8.75, 9.0, -7.75, 1.0, 1.5, 2.25, 2.5, 2.75, 3.0, 3.25, 3.5, 3.75, 4.0, 4.25, 4.5, 4.75, 5.0, 5.25, 6.25, 8.0, 10.5, 28.75, -11.25, -7.25, 1.5, 1.75, 2.0, 2.25, 2.5, 2.75, 3.0, 3.25, 3.5, 3.75, 4.0, 4.25, 4.75, 5.0, 5.25, 5.5, 5.75, 6.0, 6.25, 6.5, 7.0, 7.25, 7.5, 7.75, 14.25, 1.75, 2.0, 2.5, 3.25, 3.75, 4.0, 5.75, 6.0, 6.25, 6.5, 6.75, 7.5, 9.25, 13.0, 13.25, 14.0, 1.75, 2.0, 2.5, 3.0, 3.25, 3.5, 6.0, 8.0, 8.25, 9.25, 10.25, 13.5, 13.75, -1.75, -1.5, -1.25, 3.25, 3.5, 4.0, 7.0, 8.0, 9.0, 13.0, -9.5, -5.0, -4.5, -4.25, -4.0, -3.75, -2.0, -1.75, -1.5, -1.25, -1.0, -0.75, -0.5, -0.25, 0.0, 0.25, 6.0, 7.5, 8.75, 9.5, 10.25, 12.25, 12.5, -5.5, -5.25, -5.0, -4.75, -4.5, -4.0, -3.75, -3.5, -2.0, -1.75, -1.0, -0.25, 0.25, 1.0, 1.25, 1.5, 7.5, 10.5, 10.75, -6.75, -6.5, -6.25, -6.0, -5.75, -5.5, 1.0, 1.25, 5.75, 10.5, -7.5, -7.25, -7.0, -6.75, -6.5, -3.5, -3.25, 1.25, 10.25, -7.0, -6.75, -3.5, 9.0, -4.0, -4.25, 17.25, 17.0, 17.0, 3.0, 3.25, 16.5, 16.5, 16.75, 3.0, 13.0, 13.25, 13.5, 13.75, 14.0, 14.25, 14.5, 14.75, 15.0, 15.25, 15.25, 15.5, 15.75, 16.0, 16.25, 16.5, 4.75, 5.0, 10.25, 16.75, 17.0, 17.25, 4.25, 4.5, 4.75, 5.0, 5.25, 5.5, 5.75, 6.0, 6.25, 6.5, 10.25, 4.25, 6.5, 6.75, 7.0, 7.25, 7.5, 7.75, 8.0, 10.0, 10.0]}, {"Y"=[-1.75], "Y"=[8.75]}, {"Y"=[-23.75, -23.5, -23.5, -22.0, -21.75, -17.5, -13.0, -13.0, -12.75, -12.5, -12.25, -11.5, -10.75, -10.75, -10.5, -10.5, -10.5, -10.5, -10.25, -10.25, -10.25, -10.0, -9.75, -9.5, -9.5, -9.5, -9.25, -9.25, -9.0, -9.0, -9.0, -9.0, -8.75, -8.75, -8.75, -8.75, -8.75, -8.75, -8.75, -8.75, -8.75, -8.5, -8.5, -8.5, -8.5, -8.5, -8.5, -8.5, -8.25, -8.25, -8.25, -8.25, -8.25, -8.25, -8.25, -8.25, -8.25, -8.25, -8.25, -8.0, -8.0, -8.0, -8.0, -7.75, -7.75, -7.75, -7.75, -7.75, -7.75, -7.75, -7.75, -7.75, -7.5, -7.5, -7.5, -7.5, -7.5, -7.5, -7.5, -7.5, -7.5, -7.5, -7.5, -7.5, -7.25, -7.25, -7.25, -7.25, -7.25, -7.25, -7.25, -7.25, -7.25, -7.25, -7.25, -7.25, -7.25, -7.25, -7.0, -7.0, -7.0, -7.0, -7.0, -7.0, -7.0, -7.0, -7.0, -7.0, -6.75, -6.75, -6.75, -6.75, -6.75, -6.75, -6.75, -6.75, -6.75, -6.75, -6.75, -6.5, -6.5, -6.5, -6.5, -6.5, -6.25, -6.25, -6.25, -6.25, -6.25, -6.25, -6.25, -6.25, -6.25, -6.25, -6.25, -6.25, -6.0, -6.0, -5.75, -5.75, -5.75, -5.75, -5.75, -5.75, -5.75, -5.75, -5.75, -5.75, -5.75, -5.75, -5.75, -5.75, -5.75, -2.25, -2.25, -2.25, -2.25, -2.25, -2.25, -2.25, -2.25, -2.25, -2.25, -2.25, -2.25, -2.25, -2.25, -2.25, -2.25, -2.25, -2.25, -2.0, -2.0, -2.0, -2.0, -2.0, -2.0, -2.0, -2.0, -2.0, -2.0, -2.0, -2.0, -2.0, -2.0, -2.0, -2.0, -2.0, -2.0, -2.0, -2.0, -2.0, -2.0, -2.0, -2.0, -1.75, -1.75, -1.75, -1.75, -1.75, -1.75, -1.75, -1.75, -1.75, -1.75, -1.75, -1.75, -1.75, -1.75, -1.75, -1.75, -1.75, -1.5, -1.5, -1.5, -1.5, -1.5, -1.5, -1.5, -1.5, -1.5, -1.5, -1.5, -1.5, -1.5, -1.25, -1.25, 1.75, 1.75, 1.75, 1.75, 1.75, 1.75, 1.75, 1.75, 1.75, 1.75, 1.75, 1.75, 1.75, 2.0, 2.0, 2.0, 2.0, 2.0, 2.0, 2.0, 2.0, 2.0, 2.0, 2.25, 2.25, 2.5, 2.5, 2.5, 2.5, 2.5, 2.5, 2.75, 2.75, 2.75, 2.75, 2.75, 2.75, 2.75, 2.75, 2.75, 3.0, 3.0, 3.0, 3.0, 3.0, 3.0, 3.0, 3.0, 3.25, 3.25, 3.25, 3.25, 3.25, 3.25, 3.25, 3.25, 3.5, 3.5, 3.5, 3.5, 3.5, 3.75, 4.0, 4.0, 4.0, 4.0, 4.25, 4.25, 4.25, 4.5, 4.5, 4.5, 4.5, 4.75, 4.75, 4.75, 5.0, 5.0, 5.5, 6.5, 7.0, 7.0, 7.25, 7.5, 7.5, 7.75, 7.75, 8.0, 8.25, 8.5, 8.75, 8.75, 10.5, 10.75, 11.0, 11.0, 11.0, 11.0, 11.0, 11.0, 11.25, 11.25, 11.25, 11.25, 11.25, 11.25, 11.25, 11.25, 11.5, 11.5, 11.5, 11.5, 11.5, 11.5, 11.5, 11.5, 11.5, 11.5, 11.5, 11.5, 11.75, 11.75, 11.75, 11.75, 11.75, 12.0, 12.0, 12.0, 12.0, 12.0, 12.0, 12.0, 12.25, 12.25, 12.5, 12.75, 13.5, 13.5, 13.5, 13.5, 13.5, -2.25, -2.25, -1.75], "Y"=[24.75, 24.75, 25.0, 24.75, 24.75, 15.25, 1.0, 4.5, 20.0, 19.75, 0.5, 14.25, 14.25, 14.5, 6.0, 14.5, 14.75, 15.5, 14.75, 15.0, 15.25, 9.5, 3.5, -3.0, 3.0, 3.25, 8.25, 16.75, 0.5, 1.5, 8.25, 12.25, 1.0, 1.25, 1.5, 2.0, 2.25, 6.0, 8.0, 8.5, 12.75, -11.5, -5.75, 1.0, 2.25, 3.0, 9.0, 12.75, -13.25, -11.0, -4.5, -1.25, 3.0, 3.25, 4.0, 6.5, 8.75, 9.0, 9.25, -15.0, 8.75, 9.0, 9.25, -13.5, -8.0, -6.25, -3.0, -2.75, 1.75, 2.0, 2.25, 9.75, -11.5, -4.5, -2.75, -1.0, -0.75, 0.0, 2.0, 2.75, 3.0, 7.0, 7.25, 7.5, -14.25, -11.5, -8.5, -8.0, -4.75, -4.25, -3.25, -3.0, -0.75, 0.25, 0.75, 2.75, 3.0, 7.75, -14.75, -14.5, -11.5, -8.25, -1.5, -1.25, 1.0, 8.0, 8.25, 10.5, -11.75, 0.25, 0.5, 0.75, 1.5, 2.0, 2.25, 2.5, 6.5, 6.75, 8.25, -19.0, 0.25, 0.5, 0.75, 6.25, -5.75, -2.5, -0.25, 0.0, 0.25, 0.5, 0.75, 1.0, 1.25, 1.5, 1.75, 2.0, 5.0, 6.25, -12.25, -10.0, -5.25, -4.25, -4.0, -3.0, -0.75, -0.5, -0.25, 2.0, 2.25, 2.5, 3.75, 4.0, 5.0, -3.25, -3.0, -2.5, -2.25, 3.0, 3.25, 3.5, 3.75, 4.0, 4.25, 4.5, 4.75, 5.0, 5.25, 5.5, 6.0, 6.5, 7.25, -12.75, -10.75, -9.25, -9.0, -8.0, -7.0, -6.25, -5.5, -5.0, -4.5, -4.0, -3.5, -3.25, -3.0, -2.75, -2.5, -2.25, 3.0, 3.25, 3.5, 3.75, 4.25, 4.5, 15.25, -15.5, -12.75, -10.75, 3.5, 3.75, 4.0, 4.25, 4.5, 4.75, 5.0, 5.25, 5.75, 6.25, 6.75, 7.25, 8.0, 15.25, -12.75, -10.75, -9.25, -8.0, -7.0, -6.25, -5.75, -5.25, -5.0, -4.5, -4.25, -3.75, -3.5, -15.75, -12.75, 3.25, 3.5, 3.75, 4.0, 4.25, 4.5, 4.75, 5.0, 5.25, 5.75, 6.25, 6.75, 7.25, -13.0, -4.5, -4.25, -3.75, 6.0, 6.25, 6.75, 7.25, 8.0, 8.75, 3.75, 10.0, 4.25, 4.5, 4.75, 6.0, 7.75, 11.25, -7.0, -6.0, -5.25, 7.5, 7.75, 8.5, 9.5, 9.75, 12.75, -12.5, -12.25, -6.75, -6.0, -5.75, 8.25, 8.5, 9.25, -10.5, -8.75, -8.5, 9.0, 10.25, 10.5, 12.5, 15.25, -15.5, -15.0, -10.5, -8.75, 10.5, -3.25, -12.5, -12.25, -10.0, -6.25, -8.0, -5.5, 2.25, -9.75, -8.0, -6.25, -4.75, -12.75, -5.25, -5.0, -12.5, 1.5, 1.5, 3.75, 1.25, 5.5, 5.5, 3.5, 5.75, 1.75, 3.5, 3.5, 8.0, 3.75, -1.5, 8.25, 3.5, 3.0, 2.5, 4.0, 4.25, 4.75, 5.25, 9.25, -5.5, -3.75, -2.0, 1.75, 3.25, 3.5, 8.5, 10.75, -7.5, -5.25, 1.25, 3.0, 3.25, 3.5, 8.0, 8.5, 9.5, 9.75, 10.25, 10.5, -7.5, -5.25, 1.75, 2.0, 7.5, -4.5, -4.25, -3.75, 6.75, 8.0, 13.75, 14.0, -3.5, 13.5, 12.25, 12.5, -0.75, -0.5, -0.25, 0.0, 0.25, 8.75, 12.75, 8.75]}, {"Y"=[0.85, 0.95, 0.95, 0.6, 0.6, 0.85, 0.85, -0.85, -0.85, -0.95, -0.95, -0.6, -0.6, -0.85, -0.6, -0.6, -0.85, -0.85, 0.85, 0.85], "Y"=[-0.6, -0.6, -1.4, -1.4, -0.6, -0.6, 2.4, 2.4, -0.6, -0.6, -1.4, -1.4, -0.6, -0.6, -0.6, -1.4, -1.4, -1.6, -1.6, -1.4]}]
  out "rd":dbl
  out "bb":dbl
  out "aa":dbl
  out "xx":dbl[](array[numeric])
  out "yy":dbl[](array[numeric])
  in  "a":dbl=0.7
  out "stack":bool=TRUE
  out "track_shift":dbl[][](array[numeric])
  out "R":dbl[](array[numeric])
  out "theta":dbl[](array[numeric])
  out "RXY":dbl[](array[numeric])=[73.97207949000635, 12.402968176654849, 69.25942811748455]
  out "lw":dbl=0.4
  out "tic":u32=313769281
  out "reverse":bool
  out "map_track":dbl[][](array[numeric])=[[-0.6687401515638595, -3.551350516814976], [-1.1601880006125764, -3.4580278333550782], [-1.6512488590649952, -3.3629580799680854], [-2.1418835557610314, -3.265964418362822], [-2.6320529195405924, -3.1668700102479344], [-3.12171777924361, -3.0654980173321356], [-3.6108389637099756, -2.961671601324125], [-4.250355012057505, -2.8217269001890974], [-4.733554194697693, -2.693195492254268]]
  out "track":dbl[][](array[numeric])=[[-0.6687401515638595, -3.551350516814976], [-1.1601880006125764, -3.4580278333550782], [-1.6512488590649952, -3.3629580799680854], [-2.1418835557610314, -3.265964418362822], [-2.6320529195405924, -3.1668700102479344], [-3.12171777924361, -3.0654980173321356], [-3.6108389637099756, -2.961671601324125], [-4.250355012057505, -2.8217269001890974], [-4.733554194697693, -2.693195492254268], [-5.215089885143842, -2.558342659026822], [-5.693483406062963, -2.4115492889016945], [-6.167256080122039, -2.24719627027381], [-6.634929229988109, -2.059664491538052], [-7.095024178328142, -1.8433348410893422], [-7.546062247809149, -1.5925882073226139], [-7.98656476109811, -1.301805478632852], [-8.415053040862054, -0.9653675434148765], [-8.830048409767974, -0.5776552900636165], [-9.230072190482858, -0.133049606974057], [-9.61364570567371, 0.3740686174589265], [-9.97929027800753, 0.949318494840405], [-10.386059580111024, 1.7242186788508236], [-10.53357405922493, 2.2019628347040774], [-10.66851200140239, 2.6835902739278463], [-10.772007434080049, 3.1749262819640283], [-10.825194384694537, 3.6817961442544633], [-10.809206880682517, 4.210025146240928], [-10.705178949480636, 4.765438573365376], [-10.494244618525542, 5.353861711069529], [-10.157537915253862, 5.981119844795286], [-9.676192867102248, 6.653038259984428], [-8.946295802610212, 7.461572105302583], [-8.539313408094966, 7.752602995705581], [-8.110420661696207, 8.015244834208291], [-7.660232732059987, 8.25029468946181], [-7.189364787832295, 8.458549630117131], [-6.698431997659123, 8.640806724825243], [-6.188049530186491, 8.797863042237132], [-5.658832554060375, 8.930515651003796], [-5.11139623792681, 9.039561619776274], [-4.546355750431802, 9.12579801720561], [-3.9643262602213256, 9.190021911942688], [-3.3659229359414162, 9.233030372638604], [-2.7517609462380523, 9.25562046794435], [-2.122455459757251, 9.258589266510917], [-1.4786216451450183, 9.242733836989292], [-0.8208746710473604, 9.208851248030518], [-0.1498297061102689, 9.157738568285591], [0.5338980810202378, 9.090192866405497], [1.229693521698167, 9.007011211041284], [1.9369414472775146, 8.908990670843883], [2.6550266891122614, 8.796928314464337], [3.383334078556428, 8.671621210553642], [4.121248446963983, 8.53386642776284], [4.868154625688948, 8.384461034742866], [5.623437446085289, 8.224202100144819], [6.386481739507029, 8.053886692619635], [7.156672337308164, 7.874311880818305], [7.838146127104554, 7.70968069378327], [8.321781606815595, 7.582803343212244], [8.805290536895978, 7.45544776805299], [9.287663918083021, 7.323801011645703], [9.76789275111402, 7.18405011733063], [10.244968036726283, 7.032382128447967], [10.717880775657084, 6.864984088337955], [11.18562196864372, 6.678043040340844], [11.647182616423507, 6.4677460277968315], [12.101553719733744, 6.230280094046104], [12.547726279311707, 5.961832282428966], [12.984691295894704, 5.658589636285609], [13.411439770220039, 5.3167391989562285], [13.939637565704926, 4.818324597988705], [14.177469695018669, 4.377621822306417], [14.370305638929839, 3.9092831916317614], [14.522185803389362, 3.415790251277338], [14.637150594348116, 2.8996245465557346], [14.719240417757044, 2.363267622779441], [14.77249567956704, 1.8092010252611073], [14.800956785728996, 1.2399062993133256], [14.808664142193827, 0.6578649902486369], [14.799658154912459, 0.06555864337958095], [14.777979229835777, -0.5345311959811911]]
  out "xyhc":T2={"c_idx"=71, "xc"=-91.48037348905598, "yc"=-434.27857700428615, "hc"=-0.4484199308552679, "xc_path"=12.43286899562552}
  in  "margin":dbl
  out "vr":dbl=0.75
  out "vf":dbl=3.5
  out "vw":dbl=0.9025
  out "ymax":dbl=12.0
  out "ymin":dbl=-6.0
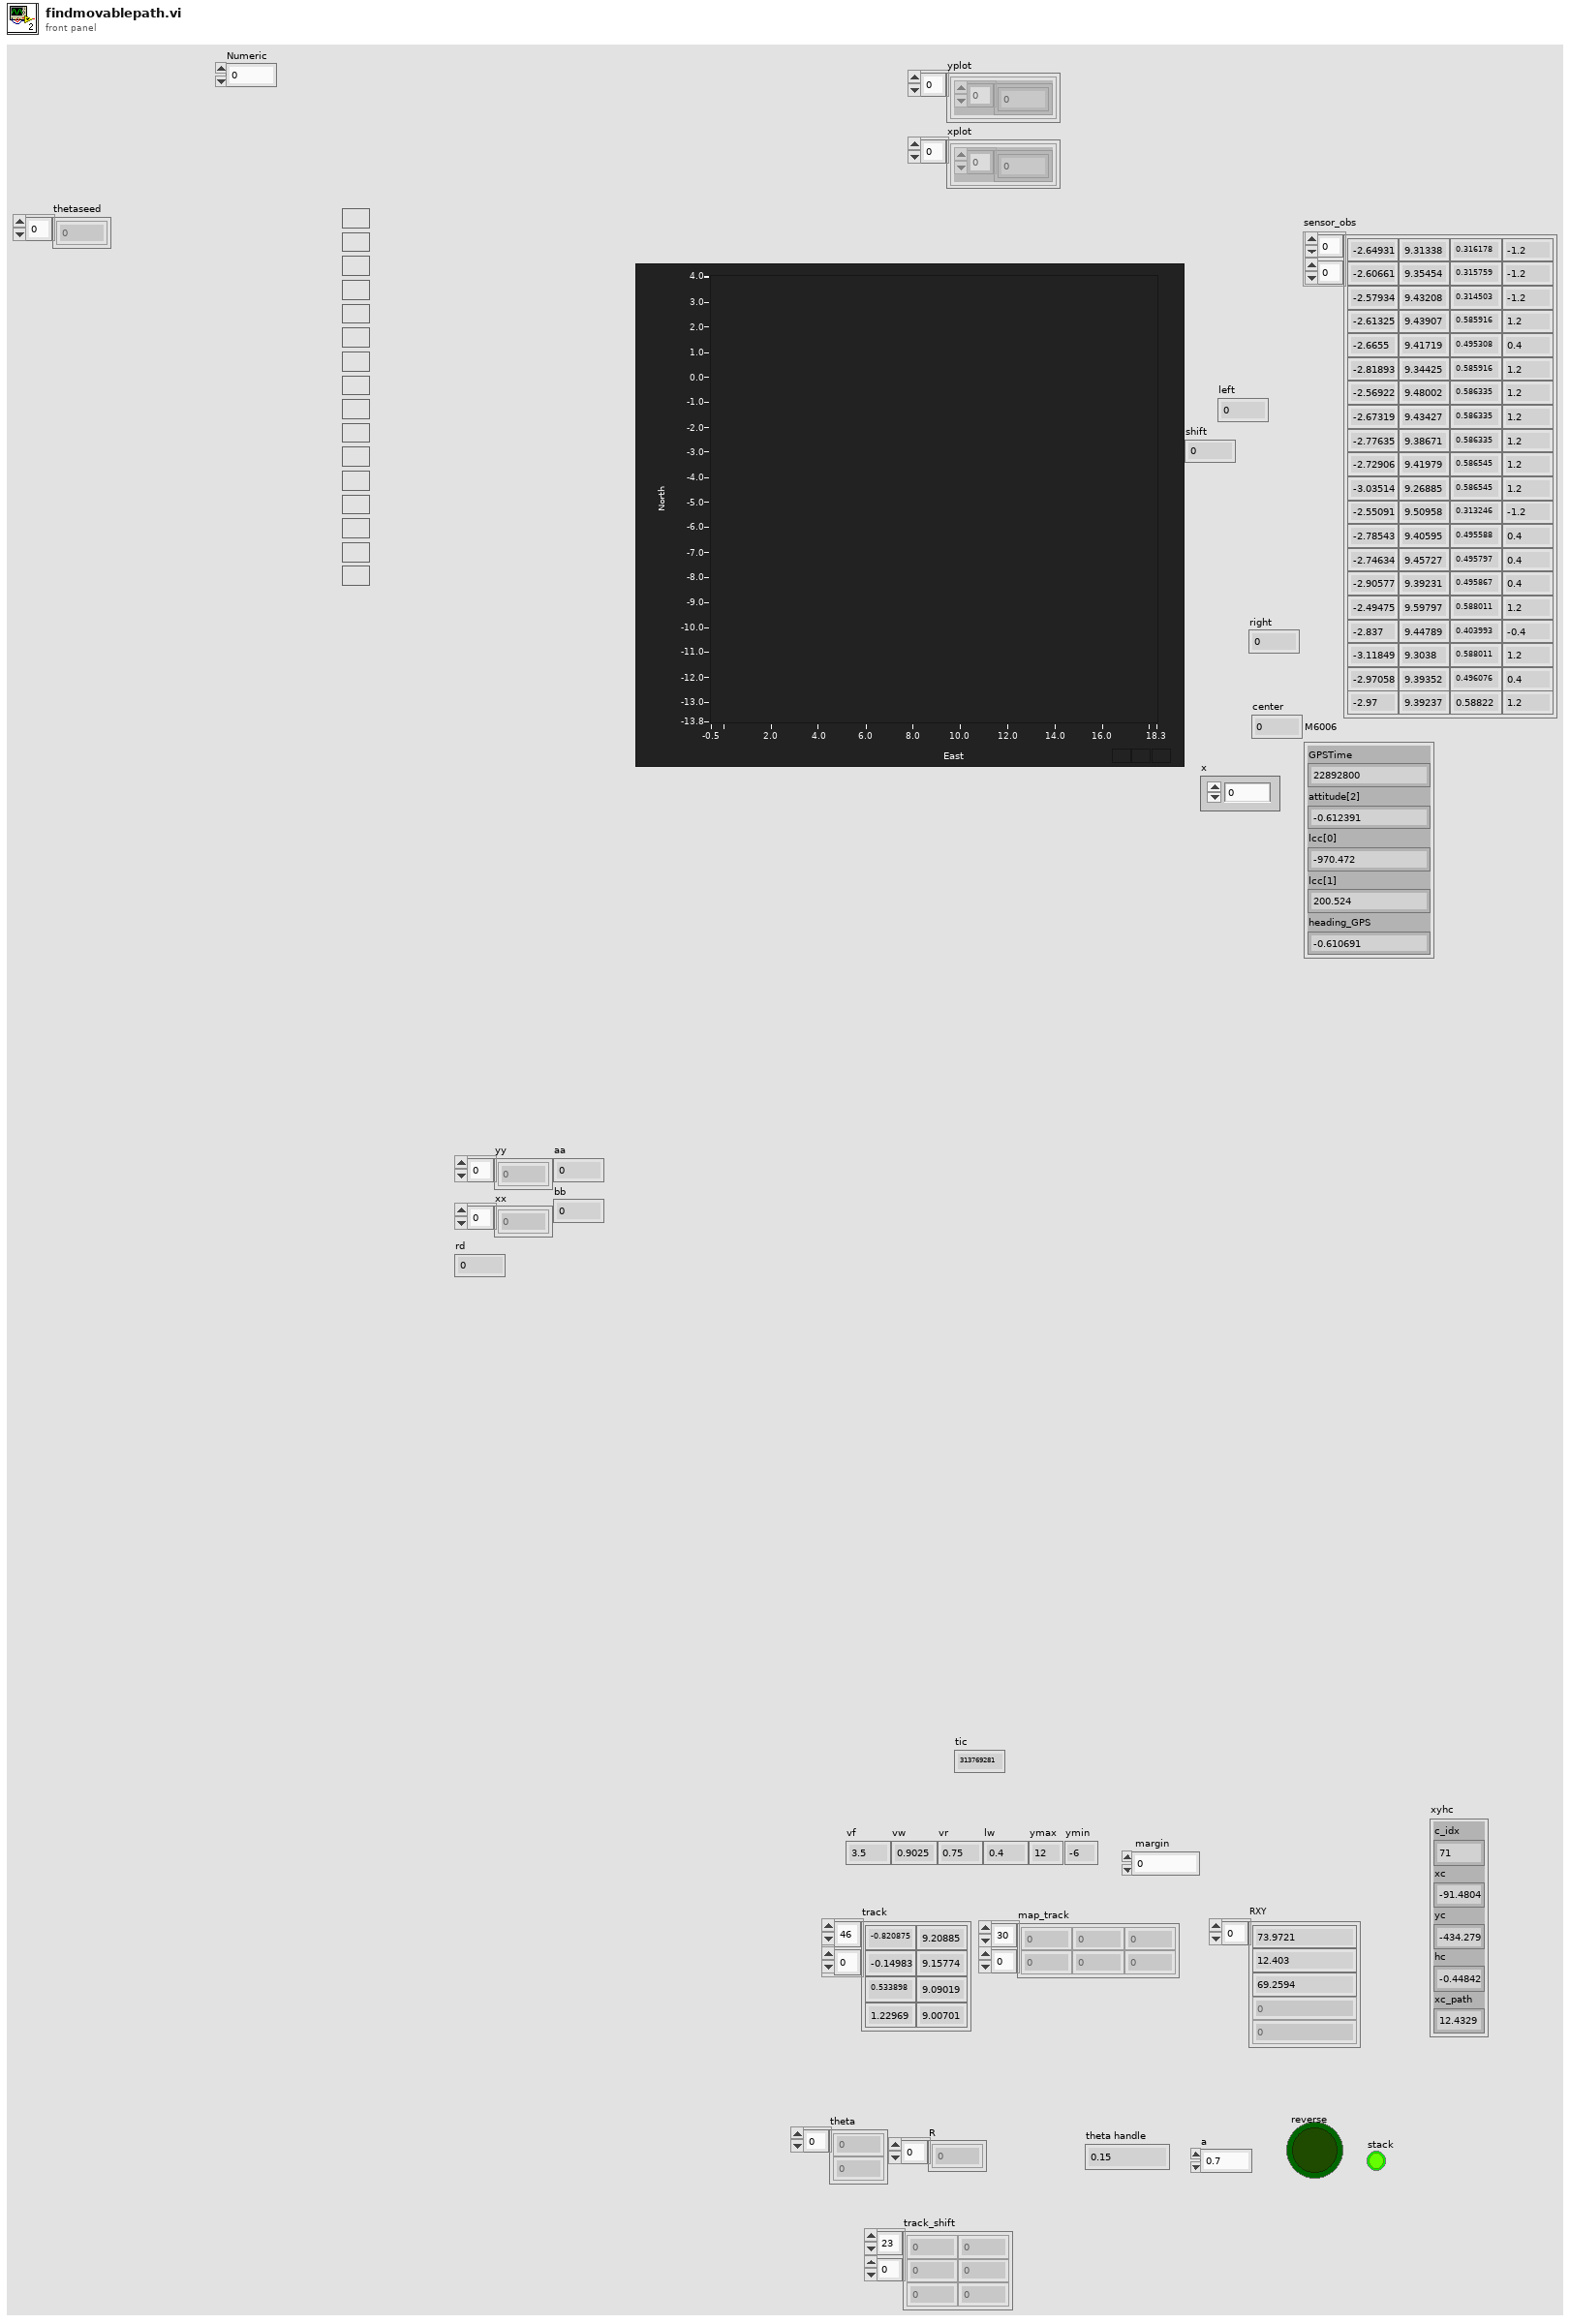
[diagram p1: front panel]
types:
  T1 = cluster{"GPSTime":dbl, "attitude[2]":sgl, "lcc[0]":sgl, "lcc[1]":sgl, "heading_GPS":sgl}
  T2 = cluster{"c_idx":i32, "xc":dbl, "yc":dbl, "hc":dbl, "xc_path":dbl}
  T3 = cluster{"GPSTime":dbl, "attitude[2]":dbl, "lcc[0]":dbl, "lcc[1]":dbl, "heading_GPS":dbl}
  T4 = cluster{"Steer_input":dbl, "Steer_output":dbl, "VS_des":dbl, "VS_can":dbl, "heading":dbl, "auto":bool, "run":bool, "x":dbl, "y":dbl}
  T5 = cluster{"idx":i32, "x":dbl, "y":dbl, "h":dbl, "x_path":dbl}
  T6 = typedef "NI_Matrix.lvlib/RealMatrix.ctl" = dbl[][]
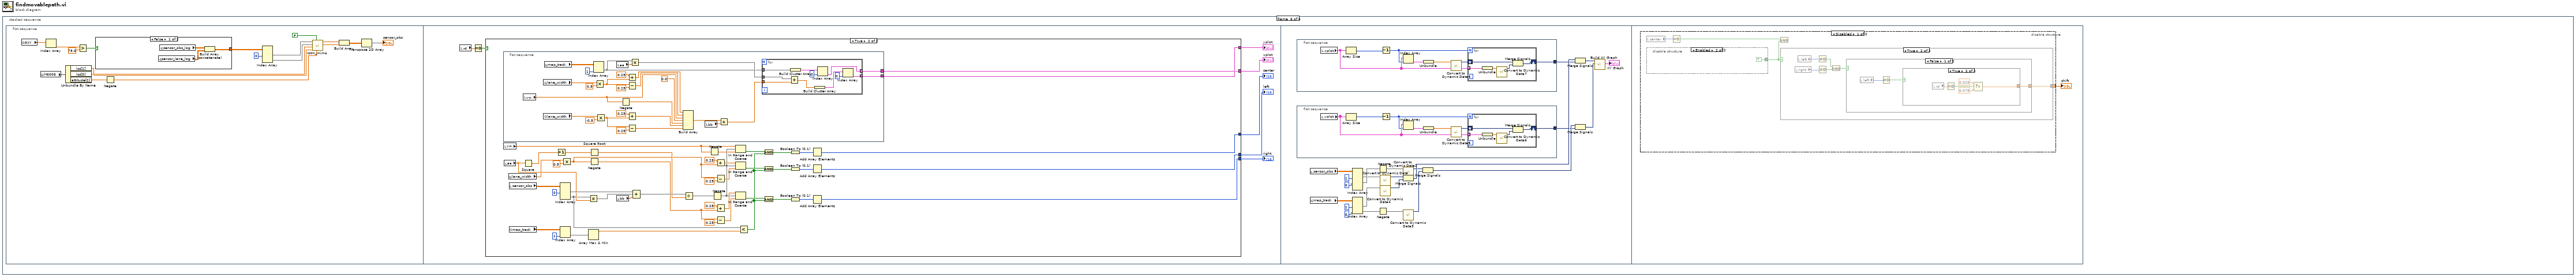
[diagram p0: block diagram]
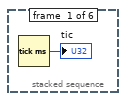
[diagram p2: hidden frame]
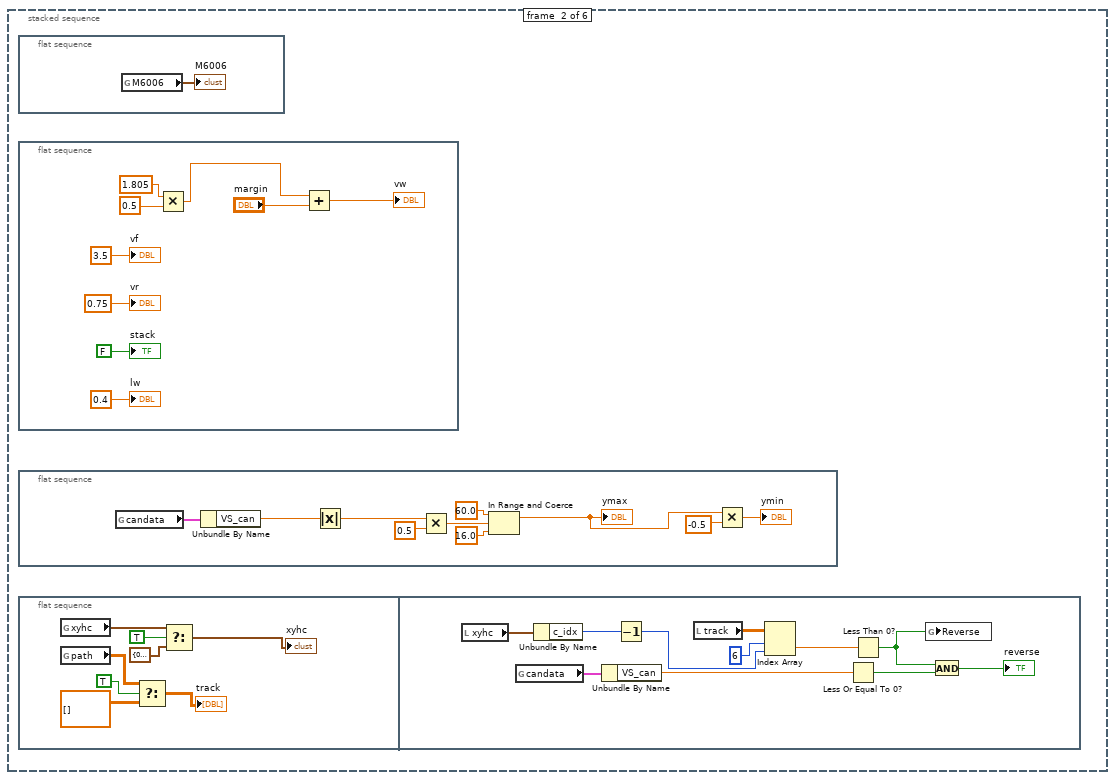
[diagram p3: hidden frame]
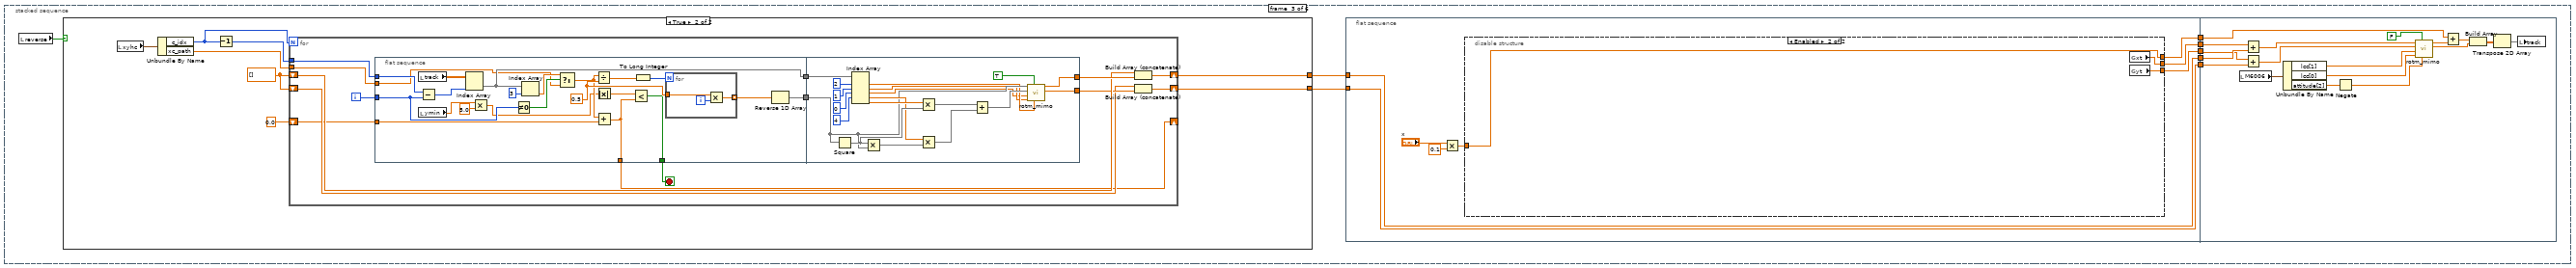
[diagram p4: hidden frame]
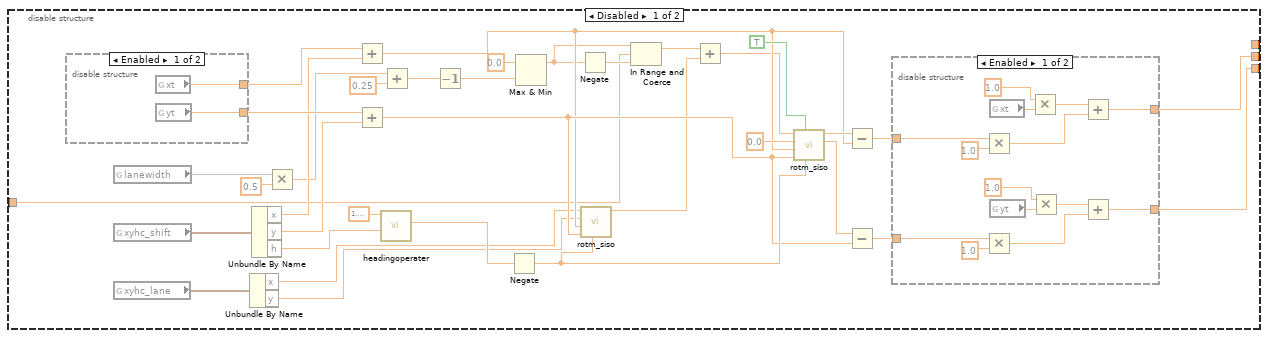
[diagram p5: hidden frame]
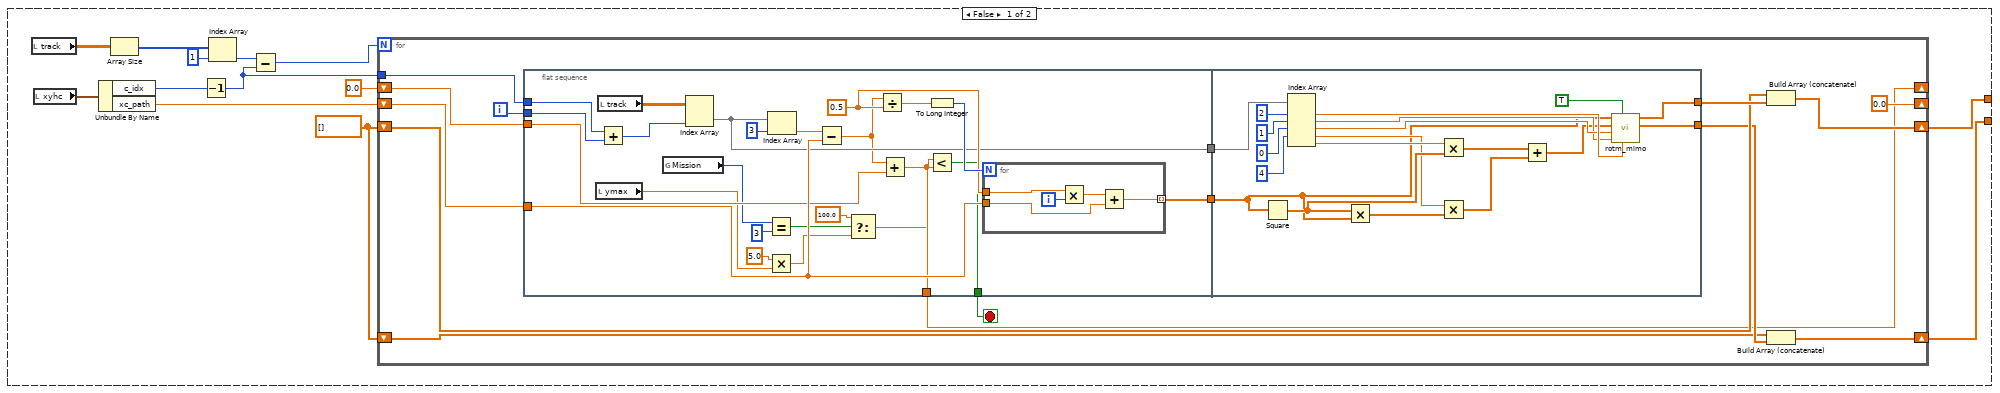
[diagram p8: hidden frame]
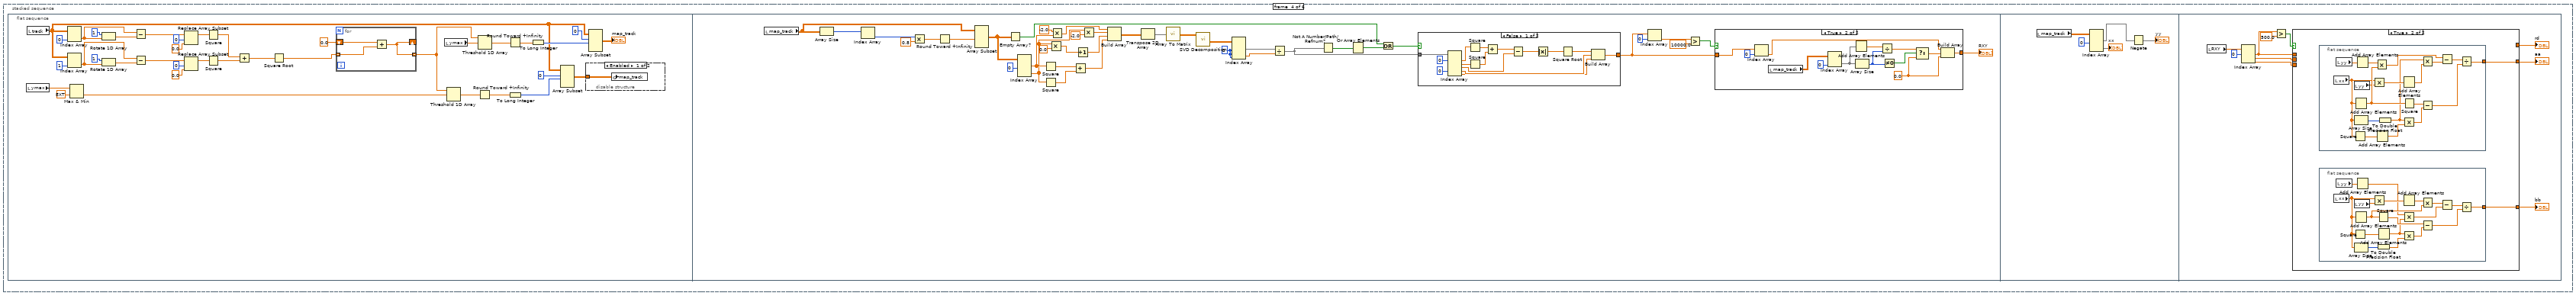
[diagram p9: hidden frame]
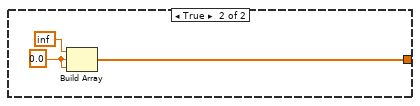
[diagram p11: hidden frame]
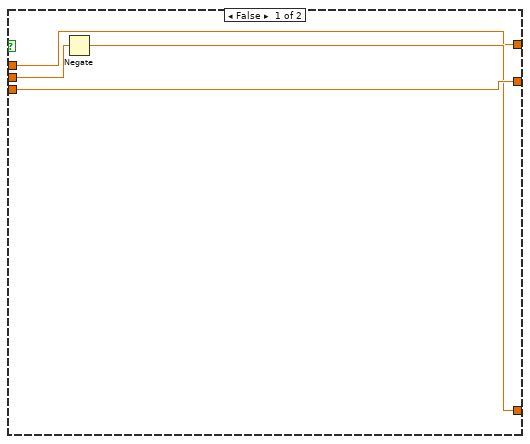
[diagram p13: hidden frame]
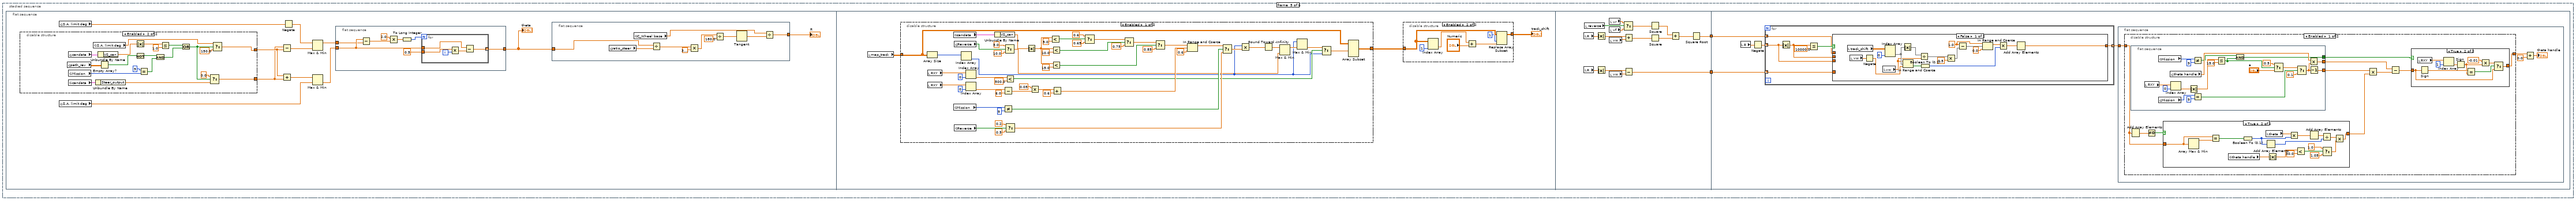
[diagram p14: hidden frame]
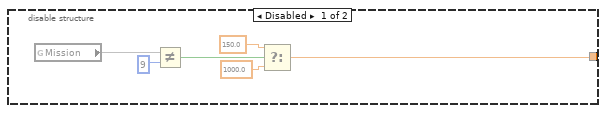
[diagram p15: hidden frame]
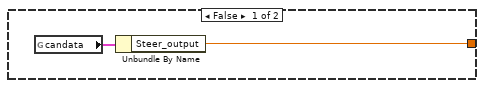
[diagram p19: hidden frame]
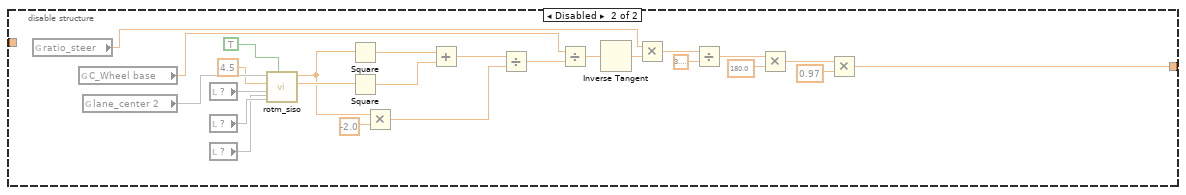
[diagram p20: hidden frame]
diagram:
  n1 = stacked-sequence {
    frame #0 {
      n2 = Tick Count (ms)() -> (millisecond timer value=→"tic":u32)
    }
    frame #1 {
      n3 = flat-sequence {
        frame #0 {
          n4 = global read "G_NAV.vi" "M6006"() -> (→"M6006":T3)
        }
      }
      n5 = flat-sequence {
        frame #0 {
          n6 = Multiply(x=1.805 ("width"), y=0.5) -> (x*y=w22:dbl)
          n7 = Add(x=w22, y="margin") -> (x+y=→"vw":dbl)
          "lw" <- 0.4 ("width")
          "vf" <- 3.5 ("af")
          "vr" <- 0.75 ("ar")
          "stack" <- FALSE
        }
      }
      n8 = flat-sequence {
        frame #0 {
          n9 = global read "G_VEH.vi" "candata"() -> (w39:T4)
          n10 = Unbundle By Name(w39) -> ("VS_can"=w36:dbl)
          n11 = Absolute Value(x=w36) -> (abs(x)=w32:dbl)
          n12 = Multiply(x=w32, y=0.5 ("vgain")) -> (x*y=w31:dbl)
          n13 = In Range and Coerce(upper limit=60.0, x=w31, lower limit=16.0 ("y")) -> (coerced(x)=w35:dbl)  [unwired: 1 out]
          "ymax" <- w35
          n14 = Multiply(x=w35, y=-0.5) -> (x*y=→"ymin":dbl)
        }
      }
      n15 = flat-sequence {
        frame #0 {
          n16 = global read "G_VEH.vi" "xyhc"() -> (w7:T5)
          n17 = global read "G_PATH.vi" "path"() -> (w2:dbl[][])
          n18 = Select(t=w2, s=TRUE ("B_track"), f=dbl[][] []) -> (s? t:f=→"track":dbl[][])
          n19 = Select(t=w7, s=TRUE ("B_track"), f=T2 {"c_idx"=0, "xc"=0.0, "yc"=0.0, "hc"=0.0, "xc_path"=0.0}) -> (s? t:f=→"xyhc":T2)
        }
        frame #1 {
          n20 = local read "xyhc"() -> (w19:T2)
          n21 = global read "G_VEH.vi" "candata"() -> (w13:T4)
          n22 = Unbundle By Name(w19) -> ("c_idx"=w17:i32)
          n23 = Unbundle By Name(w13) -> ("VS_can"=w14:dbl)
          n24 = Decrement(x=w17) -> (x-1=w18:i32)
          n25 = local read "track"() -> (w20:dbl[][])
          n26 = Index Array(array=w20, index (row)=6, index (col)=w18) -> (element=w15:dbl)
          n27 = Less Or Equal To 0?(x=w14) -> (x <= 0?=w11:bool)
          n28 = Less Than 0?(x=w15) -> (x < 0?=w12:bool)
          n29 = global write "G_VEH.vi" "Reverse"(w12) -> ()
          n30 = And(x=w12, y=w11) -> (x .and. y?=→"reverse":bool)
        }
      }
    }
    frame #2 {
      n31 = local read "reverse"() -> (w46:bool)
      n32 = case shown="True" w46 {
        tunnel: [w133 w209] -> w48
        tunnel: [w132 w208] -> w47
        frame False {
          w135 = dbl[] [] ("x")
          n33 = local read "track"() -> (w130:dbl[][])
          n34 = local read "xyhc"() -> (w129:T2)
          n35 = Unbundle By Name(w129) -> ("c_idx"=w141:i32, "xc_path"=w136:dbl)
          n36 = Array Size(array=w130) -> (size(s)=w140:i32[])
          n37 = Decrement(x=w141) -> (x-1=w137:i32)
          n38 = Index Array(array=w140, index=1) -> (element=w138:i32)
          n39 = Subtract(x=w138, y=w137) -> (x-y=w134:i32)
          n40 = for {
            N: w134 -> [_]
            tunnel: w137 -> [w155]
            shift-right: [0.0 ("xc_path")] -> _
            shift-left: w136 -> [w153]
            shift-right: [w148] -> w133
            shift-left: w135 -> [w149]
            shift-right: [w145] -> w132
            shift-left: w135 -> [w146]
            shift-right: [w143] -> _
            shift-left: 0.0 -> [w144]
            i -> [w156]
            stop <- w142 stop-if-true
            n41 = flat-sequence {
              tunnel: w156 -> [w180]
              tunnel: w155 -> [w179]
              tunnel: w153 -> [w173]
              tunnel: [w171] -> w152
              tunnel: [w170] -> w151
              tunnel: w144 -> [w168]
              tunnel: [w167] -> w143
              tunnel: [w166] -> w142
              tunnel: w152 -> [w186]
              tunnel: w151 -> [w197]
              tunnel: [w193] -> w150
              tunnel: [w192] -> w147
              frame #0 {
                w172 = 0.5 ("y")
                n42 = local read "ymax"() -> (w164:dbl)
                n43 = local read "track"() -> (w165:dbl[][])
                n44 = Add(x=w179, y=w180) -> (x+y=w178:i32)
                n45 = global read "G_PATH.vi" "Mission"() -> (w157:i32)
                n46 = Index Array(array=w165, index (col)=w178) -> (element=w170:dbl[])  [unwired: 1 in]
                n47 = Equal?(x=w157, y=3) -> (x = y?=w162:bool)
                n48 = Multiply(x=5.0 ("f"), y=w164) -> (x*y=w159:dbl)
                n49 = Index Array(array=w170, index=3) -> (element=w176:dbl)
                n50 = Subtract(x=w176, y=w173) -> (x-y=w169:dbl)
                n51 = Select(t=100.0 ("x"), s=w162, f=w159) -> (s? t:f=w158:dbl)
                n52 = Divide(x=w169, y=w172) -> (x/y=w175:dbl)
                n53 = Add(x=w169, y=w168) -> (x+y=w167:dbl)
                n54 = To Long Integer(number=w175) -> (32bit integer=w174:i32)
                n55 = Less?(x=w158, y=w167) -> (x < y?=w166:bool)
                n56 = for {
                  N: w174 -> [_]
                  tunnel: w173 -> [w181]
                  tunnel: w172 -> [w184]
                  tunnel: [w183] -> w171 mode=indexing
                  i -> [w185]
                  n57 = Multiply(x=w184, y=w185) -> (x*y=w182:dbl)
                  n58 = Add(x=w182, y=w181) -> (x+y=w183:dbl)
                }
              }
              frame #1 {
                n59 = Square(x=w186) -> (x^2=w202:dbl[])
                n60 = Index Array(array=w197, index #1=2 ("index"), index #2=1 ("index"), index #3=0 ("index"), index #4=4 ("index")) -> (element #1=w190:dbl, element #2=w188:dbl, element #3=w189:dbl, element #4=w201:dbl, element #5=w203:dbl)  [unwired: 1 in]
                n61 = Multiply(x=w202, y=w186) -> (x*y=w200:dbl[])
                n62 = Multiply(x=w203, y=w202) -> (x*y=w199:dbl[])
                n63 = Multiply(x=w201, y=w200) -> (x*y=w198:dbl[])
                n64 = Add(x=w199, y=w198) -> (x+y=w187:dbl[])
                n65 = call "rotm_mimo.vi"("angle[rad]"=w190, "reverse"=TRUE, "y0"=w188, "x0"=w189, "y"=w187, "x"=w186) -> ("Y"=w192:dbl[], "X"=w193:dbl[])  [unwired: 2 in, 2 out]
              }
            }
            n66 = Build Array (concatenate)(w149, w150) -> (w148:dbl[])
            n67 = Build Array (concatenate)(w146, w147) -> (w145:dbl[])
          }
        }
        frame True {
          w210 = dbl[] [] ("x")
          n68 = local read "xyhc"() -> (w205:T2)
          n69 = Unbundle By Name(w205) -> ("c_idx"=w207:i32, "xc_path"=w211:dbl)
          n70 = Decrement(x=w207) -> (x-1=w212:i32)
          n71 = for {
            N: w207 -> [_]
            tunnel: w212 -> [w225]
            shift-right: [w219] -> w209
            shift-left: w210 -> [w220]
            shift-right: [w216] -> w208
            shift-left: w210 -> [w217]
            tunnel: w211 -> [w224]
            shift-right: [w214] -> _
            shift-left: 0.0 -> [w215]
            i -> [w226]
            stop <- w213 stop-if-true
            n72 = flat-sequence {
              tunnel: w226 -> [w241]
              tunnel: w225 -> [w248]
              tunnel: w224 -> [w238]
              tunnel: [w236] -> w223
              tunnel: [w242] -> w222
              tunnel: w215 -> [w234]
              tunnel: [w233] -> w214
              tunnel: [w232] -> w213
              tunnel: w223 -> [w256]
              tunnel: w222 -> [w263]
              tunnel: [w259] -> w221
              tunnel: [w258] -> w218
              frame #0 {
                w243 = 0.5 ("y")
                n73 = local read "track"() -> (w231:dbl[][])
                n74 = local read "ymin"() -> (w229:dbl)
                n75 = Subtract(x=w248, y=w241) -> (x-y=w247:i32)
                n76 = Index Array(array=w231, index (col)=w247) -> (element=w242:dbl[])  [unwired: 1 in]
                n77 = Multiply(x=w229, y=5.0) -> (x*y=w228:dbl)
                n78 = Not Equal To 0?(x=w241) -> (x != 0?=w240:bool)
                n79 = Index Array(array=w242, index=3) -> (element=w239:dbl)
                n80 = Select(t=w239, s=w240, f=w238) -> (s? t:f=w235:dbl)
                n81 = Divide(x=w235, y=w243) -> (x/y=w245:dbl)
                n82 = Absolute Value(x=w228) -> (abs(x)=w230:dbl)
                n83 = Add(x=w235, y=w234) -> (x+y=w233:dbl)
                n84 = Less?(x=w230, y=w233) -> (x < y?=w232:bool)
                n85 = To Long Integer(number=w245) -> (32bit integer=w244:i32)
                n86 = for {
                  N: w244 -> [_]
                  tunnel: w243 -> [w250]
                  tunnel: [w249] -> w237 mode=indexing
                  i -> [w251]
                  n87 = Multiply(x=w250, y=w251) -> (x*y=w249:dbl)
                }
                n88 = Reverse 1D Array(array=w237) -> (reversed array=w236:dbl[])
              }
              frame #1 {
                n89 = Square(x=w256) -> (x^2=w268:dbl[])
                n90 = Index Array(array=w263, index #1=2 ("index"), index #2=1 ("index"), index #3=0 ("index"), index #4=4 ("index")) -> (element #1=w254:dbl, element #2=w253:dbl, element #3=w252:dbl, element #4=w267:dbl, element #5=w269:dbl)  [unwired: 1 in]
                n91 = Multiply(x=w268, y=w256) -> (x*y=w266:dbl[])
                n92 = Multiply(x=w269, y=w268) -> (x*y=w265:dbl[])
                n93 = Multiply(x=w267, y=w266) -> (x*y=w264:dbl[])
                n94 = Add(x=w265, y=w264) -> (x+y=w257:dbl[])
                n95 = call "rotm_mimo.vi"("angle[rad]"=w254, "reverse"=TRUE, "y0"=w253, "x0"=w252, "y"=w257, "x"=w256) -> ("Y"=w258:dbl[], "X"=w259:dbl[])  [unwired: 2 in, 2 out]
              }
            }
            n96 = Build Array (concatenate)(w220, w221) -> (w219:dbl[])
            n97 = Build Array (concatenate)(w217, w218) -> (w216:dbl[])
          }
        }
      }
      n98 = flat-sequence {
        tunnel: w47 -> [w55]
        tunnel: w48 -> [w56]
        tunnel: [w56] -> w45
        tunnel: [w55] -> w44
        tunnel: [w54] -> w43
        tunnel: [w53] -> w42
        tunnel: [w49] -> w41
        tunnel: w45 -> [w119]
        tunnel: w44 -> [w117]
        tunnel: w43 -> [w115]
        tunnel: w42 -> [w114]
        tunnel: w41 -> [w112]
        frame #0 {
          n99 = Multiply(x="x", y=0.1) -> (x*y=w50:dbl)
          n100 = disable-structure shown="Enabled" {
            disable-tunnel: [w63 w110] -> w54
            disable-tunnel: [w62 w109] -> w53
            disable-tunnel: w50 -> [w58 w108]
            disable-tunnel: [_ w108] -> w49
            frame Disabled {
              n101 = disable-structure shown="Enabled" {
                disable-tunnel: [w107 _] -> w76
                disable-tunnel: [w106 _] -> w78
                frame Enabled {
                  n102 = global read "G_PATH.vi" "xt"() -> (w107:dbl)
                  n103 = global read "G_PATH.vi" "yt"() -> (w106:dbl)
                }
                frame Disabled {
                }
              }
              n104 = global read "G_PATH.vi" "lanewidth"() -> (w69)
              n105 = global read "G_VEH.vi" "xyhc_shift"() -> (w72:T5)
              n106 = global read "G_VEH.vi" "xyhc_lane"() -> (w91:T5)
              n107 = Unbundle By Name(w91) -> ("x"=w74:dbl, "y"=w73:dbl)
              n108 = Unbundle By Name(w72) -> ("x"=w75:dbl, "y"=w77:dbl, "h"=w81:dbl)
              n109 = Multiply(x=w69, y=0.5) -> (x*y=w61:dbl)
              n110 = Add(x=w76, y=w75) -> (x+y=w83:dbl)
              n111 = Add(x=w78, y=w77) -> (x+y=w84:dbl)
              n112 = call "headingoperater.vi"("h1"=w81, "h2"=1.5707963267948966) -> ("h2-h1"=w89:dbl)  [unwired: 8 in, 1 out]
              n113 = Add(x=w61, y=0.25) -> (x+y=w59:dbl)
              n114 = Decrement(x=w59) -> (x-1=w66:dbl)
              n115 = Negate(x=w89) -> (-x=w90:dbl)
              n116 = Max & Min(x=0.0, y=w66) -> (max(x,y)=w65:dbl)  [unwired: 1 out]
              n117 = Negate(x=w65) -> (-x=w64:dbl)
              n118 = call "rotm_siso.vi"("angle[rad]"=w90, "y0"=w84, "x0"=w83, "y"=w73, "x"=w74) -> ("x'"=w71:dbl)  [unwired: 5 in, 1 out]
              n119 = In Range and Coerce(upper limit=w65, x=w58, lower limit=w64) -> (coerced(x)=w57:dbl)  [unwired: 1 out]
              n120 = Add(x=w57, y=w71) -> (x+y=w70:dbl)
              n121 = call "rotm_siso.vi"("angle[rad]"=w90, "reverse"=TRUE, "y0"=w84, "x0"=w83, "y"=0.0, "x"=w70) -> ("y'"=w87:dbl, "x'"=w86:dbl)  [unwired: 4 in]
              n122 = Subtract(x=w86, y=w83) -> (x-y=w79:dbl)
              n123 = Subtract(x=w87, y=w84) -> (x-y=w80:dbl)
              n124 = disable-structure shown="Enabled" {
                disable-tunnel: w79 -> [w101 _]
                disable-tunnel: w80 -> [w95 _]
                disable-tunnel: [w93 _] -> w63
                disable-tunnel: [w92 _] -> w62
                frame Enabled {
                  n125 = Multiply(x=w101, y=1.0 ("x")) -> (x*y=w100:dbl)
                  n126 = Multiply(x=w95, y=1.0 ("x")) -> (x*y=w94:dbl)
                  n127 = global read "G_PATH.vi" "xt"() -> (w105:dbl)
                  n128 = global read "G_PATH.vi" "yt"() -> (w98:dbl)
                  n129 = Multiply(x=1.0, y=w105) -> (x*y=w103:dbl)
                  n130 = Multiply(x=1.0, y=w98) -> (x*y=w97:dbl)
                  n131 = Add(x=w103, y=w100) -> (x+y=w93:dbl)
                  n132 = Add(x=w97, y=w94) -> (x+y=w92:dbl)
                }
                frame Disabled {
                }
              }
            }
            frame Enabled {
              n133 = global read "G_PATH.vi" "xt"() -> (w110:dbl)
              n134 = global read "G_PATH.vi" "yt"() -> (w109:dbl)
            }
          }
        }
        frame #1 {
          n135 = local read "M6006"() -> (w121:T1)
          n136 = Add(x=w115, y=w119) -> (x+y=w118:dbl[])
          n137 = Add(x=w114, y=w117) -> (x+y=w116:dbl[])
          n138 = Unbundle By Name(w121) -> ("lcc[1]"=w125:sgl, "lcc[0]"=w124:sgl, "attitude[2]"=w120:sgl)
          n139 = Negate(x=w120) -> (-x=w122:sgl)
          n140 = call "rotm_mimo.vi"("angle[rad]"=w122, "reverse"=FALSE, "y0"=w124, "x0"=w125, "y"=w116, "x"=w118) -> ("Y"=w127:dbl[], "X"=w113:dbl[])  [unwired: 2 in, 2 out]
          n141 = Add(x=w112, y=w113) -> (x+y=w111:dbl[])
          n142 = Build Array(w111, w127) -> (w126:dbl[][])
          n143 = Transpose 2D Array(2D array=w126) -> (transposed array=w128:dbl[][])
          n144 = local write "track"(w128) -> ()
        }
      }
    }
    frame #3 {
      n145 = flat-sequence {
        frame #0 {
          n146 = local read "ymax"() -> (w275:dbl)
          n147 = local read "track"() -> (w271:dbl[][])
          n148 = Index Array(array=w271, index (col)=0 ("disabled index (col)")) -> (element=w303:dbl[])  [unwired: 1 in]
          n149 = Index Array(array=w271, index (col)=1 ("disabled index (col)")) -> (element=w292:dbl[])  [unwired: 1 in]
          n150 = Max & Min(x=w275, y=ext 40.0 ("threshold y")) -> (min(x,y)=w273:ext)  [unwired: 1 out]
          n151 = Rotate 1D Array(1:w303, 2:1 ("n")) -> (0:w302:dbl[])
          n152 = Rotate 1D Array(1:w292, 2:1 ("n")) -> (0:w293:dbl[])
          n153 = Subtract(x=w303, y=w302) -> (x-y=w301:dbl[])
          n154 = Subtract(x=w292, y=w293) -> (x-y=w294:dbl[])
          n155 = Replace Array Subset(array=w301, new element=0.0 ("new element/subarray"), index=0) -> (w298:dbl[])
          n156 = Replace Array Subset(array=w294, new element=0.0 ("new element/subarray"), index=0) -> (w297:dbl[])
          n157 = Square(x=w298) -> (x^2=w289:dbl[])
          n158 = Square(x=w297) -> (x^2=w288:dbl[])
          n159 = Add(x=w289, y=w288) -> (x+y=w287:dbl[])
          n160 = Square Root(x=w287) -> (sqrt(x)=w286:dbl[])
          n161 = for {
            tunnel: w286 -> [w311] mode=indexing
            shift-right: [w309] -> _
            shift-left: 0.0 -> [w310]
            tunnel: [w309] -> w276 mode=indexing
            n162 = Add(x=w310, y=w311) -> (x+y=w309:dbl)
          }
          n163 = local read "ymax"() -> (w284:dbl)
          n164 = Threshold 1D Array(2:w273, 3:w276) -> (0:w278:dbl)  [unwired: 1 in]
          n165 = Round Toward +Infinity(x=w278) -> (ceil(x): smallest int >= x=w279:dbl)
          n166 = Threshold 1D Array(2:w284, 3:w276) -> (0:w283:dbl)  [unwired: 1 in]
          n167 = Round Toward +Infinity(x=w283) -> (ceil(x): smallest int >= x=w282:dbl)
          n168 = To Long Integer(number=w279) -> (32bit integer=w277:i32)
          n169 = To Long Integer(number=w282) -> (32bit integer=w306:i32)
          n170 = Array Subset(array=w271, index (row)=0 ("index"), length (row)=w277) -> (w272:dbl[][])  [unwired: 2 in]
          n171 = disable-structure shown="Enabled" {
            disable-tunnel: w272 -> [w308 _]
            frame Enabled {
              n172 = global write "G_PATH.vi" "map_track"(w308) -> ()
            }
            frame Disabled {
            }
          }
          n173 = Array Subset(array=w271, index (row)=0 ("index"), length (row)=w306) -> (→"map_track":dbl[][])  [unwired: 2 in]
        }
        frame #1 {
          w326 = 3 ("disabled index (col)")
          n174 = local read "map_track"() -> (w312:dbl[][])
          n175 = Array Size(array=w312) -> (size(s)=w317:i32[])
          n176 = Index Array(array=w317) -> (element=w316:i32)  [unwired: 1 in]
          n177 = Multiply(x=w316, y=0.8) -> (x*y=w314:dbl)
          n178 = Round Toward +Infinity(x=w314) -> (ceil(x): smallest int >= x=w313:dbl)
          n179 = Array Subset(array=w312, length (row)=w313) -> (w318:dbl[][])  [unwired: 3 in]
          n180 = Empty Array?(array=w318) -> (empty?=w320:bool)
          n181 = Index Array(array=w318, index (col) #1=0 ("disabled index (col)")) -> (element #1=w335:dbl[], element #2=w334:dbl[])  [unwired: 3 in]
          n182 = Square(x=w335) -> (x^2=w333:dbl[])
          n183 = Square(x=w334) -> (x^2=w332:dbl[])
          n184 = Multiply(x=w334, y=0.0) -> (x*y=w337:dbl[])
          n185 = Multiply(x=-2.0, y=w335) -> (x*y=w340:dbl[])
          n186 = Add(x=w333, y=w332) -> (x+y=w331:dbl[])
          n187 = Increment(x=w337) -> (x+1=w336:dbl[])
          n188 = Multiply(x=w334, y=-2.0) -> (x*y=w339:dbl[])
          n189 = Build Array(w340, w339, w336, w331) -> (w330:dbl[][])
          n190 = Transpose 2D Array(2D array=w330) -> (transposed array=w329:dbl[][])
          n191 = call-poly <vilib>:"Array To Matrix.vi"("Real 2D Array"=w329) -> ("Real Matrix"=w328:T6)
          n192 = call-poly <vilib>:"SVD Decomposition.vi"("A"=w328) -> ("Matrix V"=w327:T6)  [unwired: 6 in, 4 out]
          n193 = Index Array(array=w327, index (col) #1=w326, index (row) #2=w326, index (col) #2=w326) -> (element #1=w325:dbl[], element #2=w324:dbl)  [unwired: 1 in]
          n194 = Divide(x=w325, y=w324) -> (x/y=w323:dbl[])
          n195 = Not A Number/Path/Refnum?(number/path/refnum=w323) -> (NaN/Path/Refnum?=w322:bool[])
          n196 = Or Array Elements(Boolean array=w322) -> (logical OR=w321:bool)
          n197 = Or(x=w320, y=w321) -> (x .or. y?=w319:bool)
          n198 = case shown="False" w319 {
            tunnel: [w354 w365] -> w344
            tunnel: w323 -> [w350 _]
            frame False {
              n199 = Index Array(array=w350, index #1=0 ("index"), index #4=0 ("index")) -> (element #1=w363:dbl, element #2=w362:dbl, element #3=w355:dbl, element #4=w352:dbl, element #5=w351:dbl)  [unwired: 3 in]
              n200 = Square(x=w363) -> (x^2=w361:dbl)
              n201 = Square(x=w362) -> (x^2=w360:dbl)
              n202 = Add(x=w361, y=w360) -> (x+y=w356:dbl)
              n203 = Subtract(x=w356, y=w355) -> (x-y=w358:dbl)
              n204 = Absolute Value(x=w358) -> (abs(x)=w359:dbl)
              n205 = Square Root(x=w359) -> (sqrt(x)=w357:dbl)
              n206 = Build Array(w357, w352, w351) -> (w354:dbl[])
            }
            frame True {
              w367 = 0.0 ("element")
              n207 = Build Array(inf, w367, w367) -> (w365:dbl[])
            }
          }
          n208 = Index Array(array=w344, index=0) -> (element=w348:dbl)
          n209 = Greater?(x=w348, y=10000.0) -> (0:w346:bool)
          n210 = case shown="True" w346 {
            tunnel: [w368 w374] -> w345
            tunnel: w344 -> [w368 w377]
            frame False {
            }
            frame True {
              w369 = 0.0 ("element")
              n211 = Index Array(array=w377, index=0) -> (element=w375:dbl)
              n212 = local read "map_track"() -> (w381:dbl[][])
              n213 = Index Array(array=w381, index (col)=0 ("disabled index (col)")) -> (element=w379:dbl[])  [unwired: 1 in]
              n214 = Add Array Elements(numeric array=w379) -> (sum=w378:dbl)
              n215 = Array Size(array=w379) -> (size(s)=w373:i32)
              n216 = Divide(x=w378, y=w373) -> (x/y=w371:dbl)
              n217 = Not Equal To 0?(x=w373) -> (x != 0?=w372:bool)
              n218 = Select(t=w371, s=w372, f=w369) -> (s? t:f=w370:dbl)
              n219 = Build Array(w375, w370, w369) -> (w374:dbl[])
            }
          }
          "RXY" <- w345
        }
        frame #2 {
          n220 = local read "map_track"() -> (w386:dbl[][])
          n221 = Index Array(array=w386, index (col) #1=0 ("disabled index (col)")) -> (element #1=w384:dbl[], element #2=→"xx":dbl[])  [unwired: 3 in]
          n222 = Negate(x=w384) -> (-x=→"yy":dbl[])
        }
        frame #3 {
          n223 = local read "RXY"() -> (w396:dbl[])
          n224 = Index Array(array=w396, index #1=0 ("index")) -> (element #1=w387:dbl, element #2=w392:dbl, element #3=w390:dbl)  [unwired: 2 in]
          n225 = Greater?(x=w387, y=500.0) -> (0:w393:bool)
          n226 = case shown="True" w393 {
            tunnel: w392 -> [w400 _]
            tunnel: [w399 w402] -> w391
            tunnel: w390 -> [w399 _]
            tunnel: [w398 w401] -> w389
            tunnel: [w397 _] -> w388
            tunnel: w387 -> [w397 _]
            frame False {
              n227 = Negate(x=w400) -> (-x=w398:dbl)
            }
            frame True {
              n228 = flat-sequence {
                tunnel: [w405] -> w402
                frame #0 {
                  n229 = local read "xx"() -> (w406:dbl[])
                  n230 = local read "yy"() -> (w408:dbl[])
                  n231 = Square(x=w406) -> (x^2=w409:dbl[])
                  n232 = local read "yy"() -> (w407:dbl[])
                  n233 = Add Array Elements(numeric array=w406) -> (sum=w414:dbl)
                  n234 = Array Size(array=w406) -> (size(s)=w410:i32)
                  n235 = Add Array Elements(numeric array=w408) -> (sum=w413:dbl)
                  n236 = Multiply(x=w406, y=w407) -> (x*y=w415:dbl[])
                  n237 = Multiply(x=w413, y=w414) -> (x*y=w417:dbl)
                  n238 = Add Array Elements(numeric array=w409) -> (sum=w404:dbl)
                  n239 = To Double Precision Float(number=w410) -> (double precision float=w403:dbl)
                  n240 = Add Array Elements(numeric array=w415) -> (sum=w416:dbl)
                  n241 = Multiply(x=w403, y=w404) -> (x*y=w411:dbl)
                  n242 = Square(x=w414) -> (x^2=w412:dbl)
                  n243 = Multiply(x=w403, y=w416) -> (x*y=w418:dbl)
                  n244 = Subtract(x=w412, y=w411) -> (x-y=w420:dbl)
                  n245 = Subtract(x=w417, y=w418) -> (x-y=w419:dbl)
                  n246 = Divide(x=w419, y=w420) -> (x/y=w405:dbl)
                }
              }
              n247 = flat-sequence {
                tunnel: [w421] -> w401
                frame #0 {
                  n248 = local read "xx"() -> (w438:dbl[])
                  n249 = local read "yy"() -> (w436:dbl[])
                  n250 = Square(x=w438) -> (x^2=w435:dbl[])
                  n251 = local read "yy"() -> (w437:dbl[])
                  n252 = Add Array Elements(numeric array=w438) -> (sum=w431:dbl)
                  n253 = Array Size(array=w438) -> (size(s)=w434:i32)
                  n254 = Add Array Elements(numeric array=w436) -> (sum=w423:dbl)
                  n255 = Multiply(x=w438, y=w437) -> (x*y=w429:dbl[])
                  n256 = Square(x=w431) -> (x^2=w432:dbl)
                  n257 = Add Array Elements(numeric array=w435) -> (sum=w422:dbl)
                  n258 = To Double Precision Float(number=w434) -> (double precision float=w430:dbl)
                  n259 = Add Array Elements(numeric array=w429) -> (sum=w424:dbl)
                  n260 = Multiply(x=w423, y=w422) -> (x*y=w427:dbl)
                  n261 = Multiply(x=w422, y=w430) -> (x*y=w433:dbl)
                  n262 = Multiply(x=w424, y=w431) -> (x*y=w428:dbl)
                  n263 = Subtract(x=w432, y=w433) -> (x-y=w425:dbl)
                  n264 = Subtract(x=w428, y=w427) -> (x-y=w426:dbl)
                  n265 = Divide(x=w426, y=w425) -> (x/y=w421:dbl)
                }
              }
            }
          }
          "aa" <- w391
          "bb" <- w389
          "rd" <- w388
        }
      }
    }
    frame #4 {
      n266 = flat-sequence {
        tunnel: [w579] -> w440
        tunnel: [w580] -> w439
        tunnel: w440 -> [w583]
        tunnel: w439 -> [w582]
        frame #0 {
          n267 = disable-structure shown="Enabled" {
            disable-tunnel: [w453 w476] -> w442
            disable-tunnel: [_ w474] -> w441
            frame Disabled {
              n268 = global read "G_VEH.vi" "Mission"() -> (w456)
              n269 = Not Equal?(x=w456, y=9) -> (x != y?=w455:bool)
              n270 = Select(t=150.0 ("x"), s=w455, f=1000.0) -> (s? t:f=w453:dbl)
            }
            frame Enabled {
              n271 = global read "G_PATH.vi" "path_rev"() -> (w469:dbl[][])
              n272 = global read "G_VEH.vi" "candata"() -> (w477:T4)
              n273 = global read "G_PATH.vi" "Mission"() -> (w458:i32)
              n274 = global read "G_VEH.vi" "candata"() -> (w475:T4)
              n275 = global read "G_VEH.vi" "S.A. limit deg"() -> (w461:dbl)
              n276 = Unbundle By Name(w475) -> ("Steer_output"=w459:dbl)
              n277 = Unbundle By Name(w477) -> ("VS_can"=w473:dbl)
              n278 = Empty Array?(array=w469) -> (empty?=w468:bool)
              n279 = Absolute Value(x=w473) -> (abs(x)=w472:dbl)
              n280 = Not(x=w468) -> (.not. x?=w467:bool)
              n281 = Equal?(x=9 ("y"), y=w458) -> (x = y?=w466:bool)
              n282 = And(x=w467, y=w466) -> (x .and. y?=w465:bool)
              n283 = Less Or Equal?(x=w472, y=1.0) -> (x <= y?=w464:bool)
              n284 = Or(x=w464, y=w465) -> (x .or. y?=w463:bool)
              n285 = Select(t=0.0 ("f"), s=w463, f=w459) -> (s? t:f=w474:dbl)
              n286 = Select(t=w461, s=w463, f=150.0 ("t")) -> (s? t:f=w476:dbl)
            }
          }
          n287 = global read "G_VEH.vi" "S.A. limit deg"() -> (w451:dbl)
          n288 = global read "G_VEH.vi" "S.A. limit deg"() -> (w445:dbl)
          n289 = Subtract(x=w441, y=w442) -> (x-y=w443:dbl)
          n290 = Add(x=w442, y=w441) -> (x+y=w446:dbl)
          n291 = Negate(x=w451) -> (-x=w444:dbl)
          n292 = Max & Min(x=w444, y=w443) -> (max(x,y)=w447:dbl)  [unwired: 1 out]
          n293 = Max & Min(x=w446, y=w445) -> (min(x,y)=w450:dbl)  [unwired: 1 out]
          n294 = flat-sequence {
            tunnel: w450 -> [w490]
            tunnel: [w489] -> w448
            tunnel: w447 -> [w488]
            frame #0 {
              n295 = Subtract(x=w490, y=w488) -> (x-y=w495:dbl)
              n296 = Multiply(x=2.0, y=w495) -> (x*y=w493:dbl)
              n297 = To Long Integer(number=w493) -> (32bit integer=w492:i32)
              n298 = for {
                N: w492 -> [_]
                tunnel: [w499] -> w489 mode=indexing
                tunnel: 0.5 ("x") -> [w498]
                tunnel: w490 -> [w497]
                i -> [w496]
                n299 = Multiply(x=w498, y=w496) -> (x*y=w500:dbl)
                n300 = Subtract(x=w497, y=w500) -> (x-y=w499:dbl)
              }
            }
          }
          n301 = flat-sequence {
            tunnel: w448 -> [w479]
            tunnel: [w478] -> w449
            frame #0 {
              n302 = global read "G_VEH.vi" "ratio_steer"() -> (w481:dbl)
              n303 = global read "G_VEH.vi" "C_Wheel base"() -> (w486:dbl)
              n304 = Divide(x=w479, y=w481) -> (x/y=w485:dbl[])
              n305 = Multiply(x=w485, y=3.141592653589793) -> (x*y=w483:dbl[])
              n306 = Divide(x=w483, y=180.0) -> (x/y=w480:dbl[])
              n307 = Tangent(1:w480) -> (0:w487:dbl[])
              n308 = Divide(x=w486, y=w487) -> (x/y=w478:dbl[])
            }
          }
          "theta" <- w448
          "R" <- w449
        }
        frame #1 {
          n309 = local read "map_track"() -> (w503:dbl[][])
          n310 = disable-structure shown="Enabled" {
            disable-tunnel: [w564 _] -> w502
            disable-tunnel: w503 -> [w563 _]
            frame Enabled {
              n311 = Array Size(array=w563) -> (size(s)=w562:i32[])
              n312 = local read "RXY"() -> (w519:dbl[])
              n313 = local read "RXY"() -> (w556:dbl[])
              n314 = global read "G_VEH.vi" "candata"() -> (w537:T4)
              n315 = global read "G_PATH.vi" "Mission"() -> (w512:i32)
              n316 = global read "G_VEH.vi" "Reverse"() -> (w541:bool)
              n317 = global read "G_VEH.vi" "Reverse"() -> (w545:bool)
              n318 = Index Array(array=w562) -> (element=w513:i32)  [unwired: 1 in]
              n319 = Index Array(array=w519, index=0) -> (element=w518:dbl)
              n320 = Index Array(array=w556, index=0) -> (element=w553:dbl)
              n321 = Unbundle By Name(w537) -> ("VS_can"=w536:dbl)
              n322 = Subtract(x=w553, y=6.0) -> (x-y=w551:dbl)
              n323 = Not Equal?(x=w512, y=9) -> (x != y?=w546:bool)
              n324 = Select(t=5.0 ("y"), s=w541, f=10.0 ("y")) -> (s? t:f=w538:dbl)
              n325 = Less?(x=w518, y=500.0) -> (x < y?=w516:bool)
              n326 = Select(t=0.2, s=w545, f=0.5) -> (s? t:f=w542:dbl)
              n327 = Absolute Value(x=w536) -> (abs(x)=w526:dbl)
              n328 = Multiply(x=0.05, y=w551) -> (x*y=w549:dbl)
              n329 = Less?(x=w526, y=5.0) -> (x < y?=w525:bool)
              n330 = Less?(x=w526, y=10.0) -> (x < y?=w530:bool)
              n331 = Less?(x=w526, y=15.0) -> (x < y?=w534:bool)
              n332 = Add(x=w549, y=0.6 ("lower limit")) -> (x+y=w547:dbl)
              n333 = Select(t=0.6, s=w525, f=0.65 ("t")) -> (s? t:f=w522:dbl)
              n334 = Select(t=w522, s=w530, f=0.75) -> (s? t:f=w529:dbl)
              n335 = Select(t=w529, s=w534, f=0.85 ("upper limit")) -> (s? t:f=w532:dbl)
              n336 = In Range and Coerce(upper limit=w532, x=w547, lower limit=0.6) -> (coerced(x)=w521:dbl)  [unwired: 1 out]
              n337 = Select(t=w521, s=w546, f=w542) -> (s? t:f=w559:dbl)
              n338 = Multiply(x=w513, y=w559) -> (x*y=w561:dbl)
              n339 = Round Toward -Infinity(1:w561) -> (0:w558:dbl)
              n340 = Max & Min(x=w558, y=w538) -> (max(x,y)=w557:dbl)  [unwired: 1 out]
              n341 = Max & Min(x=w513, y=w557) -> (min(x,y)=w515:dbl)  [unwired: 1 out]
              n342 = Select(t=w515, s=w516, f=w513) -> (s? t:f=w514:dbl)
              n343 = Array Subset(array=w563, length (row)=w514) -> (w564:dbl[][])  [unwired: 3 in]
            }
            frame Disabled {
            }
          }
          n344 = disable-structure shown="Enabled" {
            disable-tunnel: [w504 w505] -> w501
            disable-tunnel: w502 -> [w504 w508]
            frame Disabled {
            }
            frame Enabled {
              n345 = Index Array(array=w508, index (col)=1 ("disabled index (col)")) -> (element=w510:dbl[])  [unwired: 1 in]
              n346 = Add(x=w510, y="Numeric") -> (x+y=w506:dbl[])
              n347 = Replace Array Subset(array=w508, new element=w506, index (col)=1 ("disabled index (col)")) -> (w505:dbl[][])  [unwired: 1 in]
            }
          }
          "track_shift" <- w501
        }
        frame #2 {
          n348 = local read "R"() -> (w578:dbl[])
          n349 = local read "R"() -> (w567:dbl[])
          n350 = local read "reverse"() -> (w575:bool)
          n351 = Absolute Value(x=w578) -> (abs(x)=w577:dbl[])
          n352 = Absolute Value(x=w567) -> (abs(x)=w568:dbl[])
          n353 = local read "vr"() -> (w574:dbl)
          n354 = local read "vf"() -> (w573:dbl)
          n355 = local read "vw"() -> (w566:dbl)
          n356 = local read "vw"() -> (w565:dbl)
          n357 = Select(t=w574, s=w575, f=w573) -> (s? t:f=w572:dbl)
          n358 = Add(x=w577, y=w566) -> (x+y=w576:dbl[])
          n359 = Subtract(x=w568, y=w565) -> (x-y=w580:dbl[])
          n360 = Square(x=w572) -> (x^2=w571:dbl)
          n361 = Square(x=w576) -> (x^2=w570:dbl[])
          n362 = Add(x=w571, y=w570) -> (x+y=w569:dbl[])
          n363 = Square Root(x=w569) -> (sqrt(x)=w579:dbl[])
        }
        frame #3 {
          n364 = local read "R"() -> (w585:dbl[])
          n365 = Negate(x=w585) -> (-x=w584:dbl[])
          n366 = for {
            tunnel: w584 -> [w677] mode=indexing
            tunnel: [w680] -> w581 mode=indexing
            tunnel: w583 -> [w679] mode=indexing
            tunnel: w582 -> [w678] mode=indexing
            n367 = Absolute Value(x=w677) -> (abs(x)=w676:dbl)
            n368 = Less Or Equal?(x=w676, y=10000.0) -> (x <= y?=w681:bool)
            n369 = case shown="False" w681 {
              tunnel: [w686 w701] -> w680
              tunnel: w679 -> [_ w713]
              tunnel: w678 -> [_ w718]
              tunnel: w677 -> [_ w725]
              tunnel: w676 -> [_ w712]
              frame False {
                w691 = 1.0
                n370 = local read "track_shift"() -> (w700:dbl[][])
                n371 = local read "vw"() -> (w683:dbl)
                n372 = Negate(x=w683) -> (-x=w685:dbl)
                n373 = local read "vw"() -> (w684:dbl)
                n374 = Index Array(array=w700, index (col)=0 ("disabled index (col)")) -> (element=w697:dbl[])  [unwired: 1 in]
                n375 = Absolute Value(x=w697) -> (abs(x)=w696:dbl[])
                n376 = In Range and Coerce(upper limit=w684, x=w697, lower limit=w685) -> (In Range?=w698:bool[])  [unwired: 1 out]
                n377 = Divide(x=w696, y=w684) -> (x/y=w695:dbl[])
                n378 = Boolean To (0,1)(Boolean=w698) -> (0, 1=w688:i16[])
                n379 = Multiply(x=w695, y=0.5) -> (x*y=w693:dbl[])
                n380 = Subtract(x=w691, y=w693) -> (x-y=w692:dbl[])
                n381 = In Range and Coerce(upper limit=w691, x=w692, lower limit=0.0) -> (coerced(x)=w689:dbl[])  [unwired: 1 out]
                n382 = Multiply(x=w689, y=w688) -> (x*y=w687:dbl[])
                n383 = Add Array Elements(numeric array=w687) -> (sum=w686:dbl)
              }
              frame True {
                w706 = 1.0
                n384 = Subtract(x=w713, y=w712) -> (x-y=w711:dbl)
                n385 = local read "track_shift"() -> (w728:dbl[][])
                n386 = Index Array(array=w728, index (col) #1=1 ("disabled index (col)"), index (col) #2=0 ("disabled index (col)")) -> (element #1=w722:dbl[], element #2=w726:dbl[])  [unwired: 2 in]
                n387 = Square(x=w722) -> (x^2=w721:dbl[])
                n388 = Subtract(x=w726, y=w725) -> (x-y=w724:dbl[])
                n389 = Square(x=w724) -> (x^2=w720:dbl[])
                n390 = Add(x=w721, y=w720) -> (x+y=w719:dbl[])
                n391 = Square Root(x=w719) -> (sqrt(x)=w716:dbl[])
                n392 = Subtract(x=w716, y=w712) -> (x-y=w715:dbl[])
                n393 = In Range and Coerce(upper limit=w713, x=w716, lower limit=w718) -> (In Range?=w717:bool[])  [unwired: 1 out]
                n394 = Absolute Value(x=w715) -> (abs(x)=w714:dbl[])
                n395 = Boolean To (0,1)(Boolean=w717) -> (0, 1=w703:i16[])
                n396 = Divide(x=w714, y=w711) -> (x/y=w710:dbl[])
                n397 = Multiply(x=w710, y=0.5) -> (x*y=w708:dbl[])
                n398 = Subtract(x=w706, y=w708) -> (x-y=w707:dbl[])
                n399 = In Range and Coerce(upper limit=w706, x=w707, lower limit=0.0) -> (coerced(x)=w704:dbl[])  [unwired: 1 out]
                n400 = Multiply(x=w704, y=w703) -> (x*y=w702:dbl[])
                n401 = Add Array Elements(numeric array=w702) -> (sum=w701:dbl)
              }
            }
          }
          n402 = flat-sequence {
            tunnel: w581 -> [w589]
            frame #0 {
              n403 = disable-structure shown="Enabled" {
                disable-tunnel: w589 -> [w597 _]
                disable-tunnel: [w590 w652] -> w588
                frame Enabled {
                  n404 = Add Array Elements(numeric array=w597) -> (sum=w599:dbl)
                  n405 = flat-sequence {
                    tunnel: [w618] -> w596
                    tunnel: [w617] -> w594
                    tunnel: [w609] -> w591
                    frame #0 {
                      n406 = local read "RXY"() -> (w615:dbl[])
                      n407 = global read "G_PATH.vi" "Mission"() -> (w601:i32)
                      n408 = global read "G_PATH.vi" "Mission"() -> (w600:i32)
                      n409 = global read "G_VEH.vi" "theta handle"() -> (w619:dbl)
                      n410 = Index Array(array=w615, index=0) -> (element=w613:dbl)
                      n411 = Absolute Value(x=w613) -> (abs(x)=w612:dbl)
                      n412 = Not Equal?(x=w601, y=9) -> (x != y?=w603:bool)
                      n413 = Equal?(x=w600, y=9) -> (x = y?=w607:bool)
                      n414 = Less Or Equal?(x=w612, y=15.0) -> (x <= y?=w602:bool)
                      n415 = And(x=w603, y=w602) -> (x .and. y?=w609:bool)
                      n416 = Select(t=0.5, s=w602, f="a") -> (s? t:f=w604:dbl)
                      n417 = Select(t=w604, s=w607, f=0.1) -> (s? t:f=w616:dbl)
                      n418 = Multiply(x=w619, y=w616) -> (x*y=w617:dbl)
                      n419 = Decrement(x=w616) -> (x-1=w618:dbl)
                    }
                  }
                  n420 = Not Equal To 0?(x=w599) -> (x != 0?=w598:bool)
                  n421 = case shown="True" w598 {
                    tunnel: [w632 w641] -> w595
                    tunnel: w597 -> [_ w649]
                    frame False {
                      n422 = global read "G_VEH.vi" "candata"() -> (w633:T4)
                      n423 = Unbundle By Name(w633) -> ("Steer_output"=w632:dbl)
                    }
                    frame True {
                      n424 = Array Max & Min(array=w649) -> (max value=w643:dbl)  [unwired: 3 out]
                      n425 = Equal?(x=w649, y=w643) -> (x = y?=w650:bool[])
                      n426 = global read "G_VEH.vi" "theta handle"() -> (w640:dbl)
                      n427 = Boolean To (0,1)(Boolean=w650) -> (0, 1=w645:i16[])
                      n428 = local read "theta"() -> (w644:dbl[])
                      n429 = Add Array Elements(numeric array=w645) -> (sum=w648:i16)
                      n430 = Absolute Value(x=w640) -> (abs(x)=w639:dbl)
                      n431 = Multiply(x=w644, y=w645) -> (x*y=w646:dbl[])
                      n432 = Less?(x=w639, y=30.0) -> (x < y?=w637:bool)
                      n433 = Add Array Elements(numeric array=w646) -> (sum=w647:dbl)
                      n434 = Divide(x=w647, y=w648) -> (x/y=w642:dbl)
                      n435 = Select(t=1.0, s=w637, f=1.05 ("y")) -> (s? t:f=w635:dbl)
                      n436 = Multiply(x=w642, y=w635) -> (x*y=w641:dbl)
                    }
                  }
                  n437 = Multiply(x=w596, y=w595) -> (x*y=w593:dbl)
                  n438 = Subtract(x=w594, y=w593) -> (x-y=w592:dbl)
                  n439 = case shown="True" w591 {
                    tunnel: [w621 w626] -> w590
                    tunnel: w592 -> [w621 w625]
                    frame False {
                    }
                    frame True {
                      n440 = local read "RXY"() -> (w630:dbl[])
                      n441 = Sign(1:w625) -> (0:w628:dbl)
                      n442 = Index Array(array=w630, index=1) -> (element=w629:dbl)
                      n443 = Sign(1:w629) -> (0:w624:dbl)
                      n444 = Equal?(x=w628, y=w624) -> (x = y?=w627:bool)
                      n445 = Multiply(x=-0.01, y=w624) -> (x*y=w622:dbl)
                      n446 = Select(t=w622, s=w627, f=w625) -> (s? t:f=w626:dbl)
                    }
                  }
                }
                frame Disabled {
                  n447 = global read "G_VEH.vi" "ratio_steer"() -> (w659:dbl)
                  n448 = global read "G_VEH.vi" "C_Wheel base"() -> (w662:dbl)
                  n449 = global read "G_SEN.vi" "lane_center 2"() -> (w674)
                  n450 = local read item#-1() -> (w672)
                  n451 = local read item#-1() -> (w671)
                  n452 = local read item#-1() -> (w670)
                  n453 = call "rotm_siso.vi"("angle[rad]"=w670, "reverse"=TRUE, "y0"=w671, "x0"=w672, "y"=4.5, "x"=w674) -> ("y'"=w669:dbl, "x'"=w666:dbl)  [unwired: 4 in]
                  n454 = Square(x=w666) -> (x^2=w668:dbl)
                  n455 = Square(x=w669) -> (x^2=w667:dbl)
                  n456 = Multiply(x=w666, y=-2.0) -> (x*y=w663:dbl)
                  n457 = Add(x=w668, y=w667) -> (x+y=w664:dbl)
                  n458 = Divide(x=w664, y=w663) -> (x/y=w661:dbl)
                  n459 = Divide(x=w662, y=w661) -> (x/y=w660:dbl)
                  n460 = Inverse Tangent(1:w660) -> (0:w658:dbl)
                  n461 = Multiply(x=w659, y=w658) -> (x*y=w657:dbl)
                  n462 = Divide(x=w657, y=3.141592653589793) -> (x/y=w655:dbl)
                  n463 = Multiply(x=w655, y=180.0) -> (x*y=w653:dbl)
                  n464 = Multiply(x=w653, y=0.97) -> (x*y=w652:dbl)
                }
              }
              n465 = Add(x=w588, y=0.0) -> (x+y=→"theta handle":dbl)
            }
          }
        }
      }
    }
    frame #5 {
      n466 = flat-sequence {
        frame #0 {
          n467 = global read "G_PATH.vi" "RXY"() -> (w733:dbl[])
          n468 = global read "G_NAV.vi" "M6006"() -> (w738:T3)
          n469 = Index Array(array=w733) -> (element=w732:dbl)  [unwired: 1 in]
          n470 = Unbundle By Name(w738) -> ("lcc[1]"=w743:dbl, "lcc[0]"=w742:dbl, "attitude[2]"=w744:dbl)
          n471 = Greater?(x=w732, y=75.0) -> (0:w730:bool)
          n472 = case shown="False" w730 {
            tunnel: [w747 w750] -> w729
            frame False {
              n473 = global read "G_SEN.vi" "sensor_lane_log"() -> (w748:dbl[][])
              n474 = global read "G_SEN.vi" "sensor_obs_log"() -> (w749:dbl[][])
              n475 = Build Array (concatenate)(w749, w748) -> (w747:dbl[][])
            }
            frame True {
              n476 = global read "G_SEN.vi" "sensor_obs_log"() -> (w750:dbl[][])
            }
          }
          n477 = Negate(x=w744) -> (-x=w741:dbl)
          n478 = Index Array(array=w729, index (col) #1=0 ("disabled index (col)")) -> (element #1=w745:dbl[], element #2=w746:dbl[])  [unwired: 3 in]
          n479 = call "rotm_mimo.vi"("angle[rad]"=w741, "reverse"=FALSE, "y0"=w742, "x0"=w743, "y"=w746, "x"=w745) -> ("Y"=w736:dbl[], "X"=w737:dbl[])  [unwired: 2 in, 2 out]
          n480 = Build Array(w737, w736) -> (w735:dbl[][])
          n481 = Transpose 2D Array(2D array=w735) -> (transposed array=→"sensor_obs":dbl[][])
        }
        frame #1 {
          n482 = local read "rd"() -> (w757:dbl)
          n483 = Equal To 0?(x=w757) -> (x = 0?=w756:bool)
          n484 = case shown="True" w756 {
            tunnel: [w769 w910] -> w755
            tunnel: [w771 w909] -> w754
            tunnel: [w767 w908] -> w753
            tunnel: [w761 w904] -> w751
            tunnel: [w760 w905] -> w752
            frame False {
              n485 = flat-sequence {
                tunnel: [w850] -> w762
                tunnel: w762 -> [w882]
                tunnel: [w881] -> w760
                tunnel: [w880] -> w761
                frame #0 {
                  n486 = global read "G_PATH.vi" "map_track"() -> (w835:dbl[][])
                  n487 = Index Array(array=w835, index (col) #1=1 ("disabled index (col)"), index (col) #2=0 ("index (col)")) -> (element #1=w837:dbl[], element #2=w843:dbl[])  [unwired: 2 in]
                  n488 = local read "aa"() -> (w836:dbl)
                  n489 = Negate(x=w843) -> (-x=w841:dbl[])
                  n490 = Subtract(x=w837, y=w836) -> (x-y=w840:dbl[])
                  n491 = local read "bb"() -> (w842:dbl)
                  n492 = Subtract(x=w841, y=w842) -> (x-y=w839:dbl[])
                  n493 = Re/Im To Polar(2:w839, 3:w840) -> (0:→"thetaseed":dbl[])  [unwired: 1 out]
                }
                frame #1 {
                  n494 = global read "G_PATH.vi" "lane_width"() -> (w874:dbl)
                  n495 = global read "G_PATH.vi" "lane_width"() -> (w861:dbl)
                  n496 = local read "rd"() -> (w855:dbl)
                  n497 = local read "vw"() -> (w856:dbl)
                  n498 = local read "rd"() -> (w858:dbl)
                  n499 = local read "vw"() -> (w859:dbl)
                  n500 = local read "vf"() -> (w853:dbl)
                  n501 = Add(x=w855, y=w856) -> (x+y=w854:dbl)
                  n502 = Square(x=w853) -> (x^2=w851:dbl)
                  n503 = Subtract(x=w858, y=w859) -> (x-y=w847:dbl)
                  n504 = Square(x=w854) -> (x^2=w852:dbl)
                  n505 = Multiply(x=w861, y=0.5) -> (x*y=w864:dbl)
                  n506 = Multiply(x=w874, y=-0.5) -> (x*y=w871:dbl)
                  n507 = local read "rd"() -> (w872:dbl)
                  n508 = local read "rd"() -> (w863:dbl)
                  n509 = Add(x=w852, y=w851) -> (x+y=w857:dbl)
                  n510 = Add(x=w872, y=w871) -> (x+y=w868:dbl)
                  n511 = Add(x=w863, y=w864) -> (x+y=w867:dbl)
                  n512 = Square Root(x=w857) -> (sqrt(x)=w860:dbl)
                  n513 = Subtract(x=w868, y=0.25) -> (x-y=w875:dbl)
                  n514 = Add(x=w868, y=0.25) -> (x+y=w876:dbl)
                  n515 = Subtract(x=w867, y=0.25) -> (x-y=w848:dbl)
                  n516 = Add(x=w867, y=0.25) -> (x+y=w849:dbl)
                  n517 = local read "rd"() -> (w846:dbl)
                  n518 = Build Array(w875, w876, w860, w846, w847, w848, w849) -> (w850:dbl[])
                }
                frame #2 {
                  n519 = local read "thetaseed"() -> (w879:dbl[])
                  n520 = Sine & Cosine(0:w879) -> (1:w878:dbl[], 2:w877:dbl[])
                  n521 = for {
                    tunnel: w882 -> [w893] mode=indexing
                    tunnel: [w889] -> w881 mode=indexing
                    tunnel: [w885] -> w880 mode=indexing
                    tunnel: w878 -> [w884]
                    tunnel: w877 -> [w883]
                    n522 = Multiply(x=w893, y=w884) -> (x*y=w895:dbl[])
                    n523 = Multiply(x=w893, y=w883) -> (x*y=w897:dbl[])
                    n524 = local read "bb"() -> (w894:dbl)
                    n525 = local read "aa"() -> (w896:dbl)
                    n526 = Add(x=w897, y=w896) -> (x+y=w887:dbl[])
                    n527 = Add(x=w894, y=w895) -> (x+y=w892:dbl[])
                    n528 = Build Cluster Array(w892) -> (w891:cluster{dbl[]}[])
                    n529 = Build Cluster Array(w887) -> (w886:cluster{dbl[]}[])
                    n530 = Index Array(array=w891, index=0) -> (element=w889:cluster{dbl[]})
                    n531 = Index Array(array=w886, index=0) -> (element=w885:cluster{dbl[]})
                  }
                }
              }
              n532 = global read "G_PATH.vi" "lane_width"() -> (w823:dbl)
              n533 = global read "G_PATH.vi" "lane_width"() -> (w797:dbl)
              n534 = local read "sensor_obs"() -> (w759:dbl[][])
              n535 = global read "G_PATH.vi" "map_track"() -> (w758:dbl[][])
              n536 = local read "rd"() -> (w782:dbl)
              n537 = local read "vw"() -> (w783:dbl)
              n538 = local read "rd"() -> (w786:dbl)
              n539 = local read "vw"() -> (w784:dbl)
              n540 = local read "bb"() -> (w770:dbl)
              n541 = local read "vf"() -> (w780:dbl)
              n542 = Square(x=w780) -> (x^2=w778:dbl)
              n543 = Greater Than 0?(x=w770) -> (x > 0?=w765:bool)
              n544 = Add(x=w782, y=w783) -> (x+y=w781:dbl)
              n545 = Subtract(x=w786, y=w784) -> (x-y=w785:dbl)
              n546 = Square(x=w781) -> (x^2=w779:dbl)
              n547 = Index Array(array=w759, index (col) #1=1 ("disabled index (col)"), index (col) #2=0 ("index (col)")) -> (element #1=w764:dbl[], element #2=w792:dbl[])  [unwired: 2 in]
              n548 = Index Array(array=w758, index (col) #1=1 ("disabled index (col)"), index (col) #2=0 ("index (col)")) -> (element #1=w814:dbl[], element #2=w813:dbl[])  [unwired: 2 in]
              n549 = Multiply(x=w797, y=0.5) -> (x*y=w800:dbl)
              n550 = Multiply(x=w823, y=-0.5) -> (x*y=w820:dbl)
              n551 = local read "aa"() -> (w763:dbl)
              n552 = local read "rd"() -> (w821:dbl)
              n553 = local read "rd"() -> (w799:dbl)
              n554 = Add(x=w779, y=w778) -> (x+y=w777:dbl)
              n555 = Square(x=w764) -> (x^2=w790:dbl[])
              n556 = Square(x=w792) -> (x^2=w789:dbl[])
              n557 = Square(x=w814) -> (x^2=w812:dbl[])
              n558 = Square(x=w813) -> (x^2=w811:dbl[])
              n559 = Negate(x=w792) -> (-x=w832:dbl[])
              n560 = Add(x=w821, y=w820) -> (x+y=w819:dbl)
              n561 = Add(x=w799, y=w800) -> (x+y=w801:dbl)
              n562 = Subtract(x=w764, y=w763) -> (x-y=w830:dbl[])
              n563 = local read "bb"() -> (w831:dbl)
              n564 = Add(x=w790, y=w789) -> (x+y=w791:dbl[])
              n565 = Add(x=w812, y=w811) -> (x+y=w810:dbl[])
              n566 = Subtract(x=w832, y=w831) -> (x-y=w829:dbl[])
              n567 = Square Root(x=w791) -> (sqrt(x)=w788:dbl[])
              n568 = Square Root(x=w810) -> (sqrt(x)=w809:dbl[])
              n569 = Add(x=0.25, y=w819) -> (x+y=w818:dbl)
              n570 = Add(x=0.25, y=w801) -> (x+y=w802:dbl)
              n571 = Subtract(x=w801, y=0.25) -> (x-y=w803:dbl)
              n572 = Array Max & Min(array=w809) -> (max value=w808:dbl)  [unwired: 3 out]
              n573 = Square(x=w830) -> (x^2=w828:dbl[])
              n574 = Square(x=w829) -> (x^2=w827:dbl[])
              n575 = Add(x=w828, y=w827) -> (x+y=w826:dbl[])
              n576 = Less?(x=w788, y=w808) -> (x < y?=w772:bool[])
              n577 = Square Root(x=w777) -> (sqrt(x)=w776:dbl)
              n578 = Square Root(x=w826) -> (sqrt(x)=w787:dbl[])
              n579 = Subtract(x=w819, y=0.25) -> (x-y=w817:dbl)
              n580 = In Range and Coerce(upper limit=w776, x=w787, lower limit=w785) -> (In Range?=w773:bool[])  [unwired: 1 out]
              n581 = In Range and Coerce(upper limit=w818, x=w787, lower limit=w817) -> (In Range?=w807:bool[])  [unwired: 1 out]
              n582 = In Range and Coerce(upper limit=w802, x=w787, lower limit=w803) -> (In Range?=w804:bool[])  [unwired: 1 out]
              n583 = And(x=w773, y=w772) -> (x .and. y?=w774:bool[])
              n584 = And(x=w807, y=w772) -> (x .and. y?=w806:bool[])
              n585 = And(x=w804, y=w772) -> (x .and. y?=w793:bool[])
              n586 = Boolean To (0,1)(Boolean=w774) -> (0, 1=w775:i16[])
              n587 = Boolean To (0,1)(Boolean=w806) -> (0, 1=w805:i16[])
              n588 = Boolean To (0,1)(Boolean=w793) -> (0, 1=w794:i16[])
              n589 = Add Array Elements(numeric array=w775) -> (sum=w771:i16)
              n590 = Add Array Elements(numeric array=w805) -> (sum=w768:i16)
              n591 = Add Array Elements(numeric array=w794) -> (sum=w766:i16)
              n592 = case shown="True" w765 {
                tunnel: [w898 w901] -> w769
                tunnel: w768 -> [w899 w901]
                tunnel: [w899 w900] -> w767
                tunnel: w766 -> [w898 w900]
                frame False {
                }
                frame True {
                }
              }
            }
            frame True {
              n593 = flat-sequence {
                tunnel: [w952] -> w905
                tunnel: [w951] -> w904
                frame #0 {
                  n594 = local read "vw"() -> (w966:dbl)
                  n595 = global read "G_PATH.vi" "lane_width"() -> (w971:dbl)
                  n596 = global read "G_PATH.vi" "lane_width"() -> (w961:dbl)
                  n597 = global read "G_PATH.vi" "map_track"() -> (w948:dbl[][])
                  n598 = Index Array(array=w948, index (col)=1 ("disabled index (col)")) -> (element=w949:dbl[])  [unwired: 1 in]
                  n599 = Multiply(x=w971, y=0.5) -> (x*y=w970:dbl)
                  n600 = Multiply(x=w961, y=-0.5) -> (x*y=w962:dbl)
                  n601 = local read "aa"() -> (w954:dbl)
                  n602 = Negate(x=w966) -> (-x=w965:dbl)
                  n603 = Add(x=0.25, y=w970) -> (x+y=w969:dbl)
                  n604 = Subtract(x=w970, y=0.25) -> (x-y=w968:dbl)
                  n605 = Add(x=0.25, y=w962) -> (x+y=w957:dbl)
                  n606 = Subtract(x=w962, y=0.25) -> (x-y=w956:dbl)
                  n607 = Multiply(x=w949, y=w954) -> (x*y=w950:dbl[])
                  n608 = Build Array(w969, w968, w966, 0.0 ("element"), w965, w957, w956) -> (w964:dbl[])
                  n609 = local read "bb"() -> (w963:dbl)
                  n610 = Add(x=w964, y=w963) -> (x+y=w953:dbl[])
                  n611 = for {
                    tunnel: w953 -> [w977] mode=indexing
                    tunnel: [w981] -> w952 mode=indexing
                    tunnel: [w978] -> w951 mode=indexing
                    tunnel: w950 -> [w976]
                    tunnel: w949 -> [w975]
                    n612 = Add(x=w976, y=w977) -> (x+y=w984:dbl[])
                    n613 = Build Cluster Array(w975) -> (w979:cluster{"map_track":dbl[]}[])
                    n614 = Build Cluster Array(w984) -> (w983:cluster{dbl[]}[])
                    n615 = Index Array(array=w979, index=0) -> (element=w978:cluster{"map_track":dbl[]})
                    n616 = Index Array(array=w983, index=0) -> (element=w981:cluster{dbl[]})
                  }
                }
              }
              n617 = local read "vw"() -> (w906:dbl)
              n618 = local read "aa"() -> (w943:dbl)
              n619 = global read "G_PATH.vi" "lane_width"() -> (w940:dbl)
              n620 = local read "sensor_obs"() -> (w903:dbl[][])
              n621 = global read "G_PATH.vi" "map_track"() -> (w902:dbl[][])
              n622 = Square(x=w943) -> (x^2=w936:dbl)
              n623 = Increment(x=w936) -> (x+1=w935:dbl)
              n624 = Index Array(array=w903, index (col) #1=0 ("disabled index (col)")) -> (element #1=w945:dbl[], element #2=w928:dbl[])  [unwired: 3 in]
              n625 = Index Array(array=w902, index (col)=1 ("disabled index (col)")) -> (element=w930:dbl[])  [unwired: 1 in]
              n626 = Multiply(x=w940, y=0.5) -> (x*y=w921:dbl)
              n627 = Multiply(x=w928, y=w943) -> (x*y=w944:dbl[])
              n628 = Array Max & Min(array=w930) -> (max value=w929:dbl)  [unwired: 3 out]
              n629 = Square Root(x=w935) -> (sqrt(x)=w941:dbl)
              n630 = Negate(x=w921) -> (-x=w922:dbl)
              n631 = local read "bb"() -> (w942:dbl)
              n632 = Compound Arithmetic op=ADD(w945, w944, w942) -> (w946:dbl[])
              n633 = Divide(x=w946, y=w941) -> (x/y=w937:dbl[])
              n634 = Negate(x=w906) -> (-x=w907:dbl)
              n635 = Negate(x=w937) -> (-x=w915:dbl[])
              n636 = Add(x=0.25, y=w921) -> (x+y=w932:dbl)
              n637 = Subtract(x=w921, y=0.25) -> (x-y=w917:dbl)
              n638 = Add(x=0.25, y=w922) -> (x+y=w916:dbl)
              n639 = Subtract(x=w922, y=0.25) -> (x-y=w925:dbl)
              n640 = In Range and Coerce(upper limit=w906, x=w915, lower limit=w907) -> (In Range?=w914:bool[])  [unwired: 1 out]
              n641 = In Range and Coerce(upper limit=w932, x=w915, lower limit=w917) -> (In Range?=w927:bool[])  [unwired: 1 out]
              n642 = In Range and Coerce(upper limit=w916, x=w915, lower limit=w925) -> (In Range?=w920:bool[])  [unwired: 1 out]
              n643 = Less?(x=w928, y=w929) -> (x < y?=w913:bool[])
              n644 = And(x=w914, y=w913) -> (x .and. y?=w911:bool[])
              n645 = And(x=w927, y=w913) -> (x .and. y?=w926:bool[])
              n646 = And(x=w920, y=w913) -> (x .and. y?=w918:bool[])
              n647 = Boolean To (0,1)(Boolean=w911) -> (0, 1=w912:i16[])
              n648 = Boolean To (0,1)(Boolean=w926) -> (0, 1=w938:i16[])
              n649 = Boolean To (0,1)(Boolean=w918) -> (0, 1=w919:i16[])
              n650 = Add Array Elements(numeric array=w912) -> (sum=w909:i16)
              n651 = Add Array Elements(numeric array=w938) -> (sum=w910:i16)
              n652 = Add Array Elements(numeric array=w919) -> (sum=w908:i16)
            }
          }
          "left" <- w755
          "right" <- w753
          "center" <- w754
          "yplot" <- w752
          "xplot" <- w751
        }
        frame #2 {
          n653 = flat-sequence {
            tunnel: [w1026] -> w988
            frame #0 {
              n654 = local read "xplot"() -> (w1024:cluster{dbl[]}[])
              n655 = Array Size(array=w1024) -> (size(s)=w1025:i32)
              n656 = Decrement(x=w1025) -> (x-1=w1020:i32)
              n657 = Index Array(array=w1024, index=w1020) -> (element=w1023:cluster{dbl[]})
              n658 = Unbundle(w1023) -> (w1022:dbl[])
              n659 = call "Convert to Dynamic Data5"("Array"=w1022) -> ("Dynamic Data Type"=w1021:dynamicdata)  [unwired: 3 in]
              n660 = for {
                N: w1020 -> [_]
                tunnel: w1024 -> [w1031] mode=indexing
                shift-right: [w1028] -> w1026
                shift-left: w1021 -> [w1027]
                n661 = Unbundle(w1031) -> (w1030:dbl[])
                n662 = call "Convert to Dynamic Data7"("Array"=w1030) -> ("Dynamic Data Type"=w1029:dynamicdata)  [unwired: 3 in]
                n663 = Merge Signals(w1027, w1029) -> (w1028:dynamicdata)
              }
            }
          }
          n664 = flat-sequence {
            tunnel: [w1014] -> w987
            frame #0 {
              n665 = local read "yplot"() -> (w1012:cluster{dbl[]}[])
              n666 = Array Size(array=w1012) -> (size(s)=w1013:i32)
              n667 = Decrement(x=w1013) -> (x-1=w1008:i32)
              n668 = Index Array(array=w1012, index=w1008) -> (element=w1011:cluster{dbl[]})
              n669 = Unbundle(w1011) -> (w1010:dbl[])
              n670 = call "Convert to Dynamic Data9"("Array"=w1010) -> ("Dynamic Data Type"=w1009:dynamicdata)  [unwired: 3 in]
              n671 = for {
                N: w1008 -> [_]
                tunnel: w1012 -> [w1019] mode=indexing
                shift-right: [w1016] -> w1014
                shift-left: w1009 -> [w1015]
                n672 = Unbundle(w1019) -> (w1018:dbl[])
                n673 = call "Convert to Dynamic Data6"("Array"=w1018) -> ("Dynamic Data Type"=w1017:dynamicdata)  [unwired: 3 in]
                n674 = Merge Signals(w1015, w1017) -> (w1016:dynamicdata)
              }
            }
          }
          n675 = local read "sensor_obs"() -> (w986:dbl[][])
          n676 = global read "G_PATH.vi" "map_track"() -> (w985:dbl[][])
          n677 = Index Array(array=w986, index (col) #1=1 ("disabled index (col)"), index (col) #2=0 ("index (col)")) -> (element #1=w996:dbl[], element #2=w997:dbl[])  [unwired: 4 in, 1 out]
          n678 = Index Array(array=w985, index (col) #1=1 ("disabled index (col)"), index (col) #2=0 ("index (col)")) -> (element #1=w1006:dbl[], element #2=w1001:dbl[])  [unwired: 2 in]
          n679 = Negate(x=w997) -> (-x=w998:dbl[])
          n680 = Negate(x=w1001) -> (-x=w1003:dbl[])
          n681 = call "Convert to Dynamic Data"("Array"=w996) -> ("Dynamic Data Type"=w992:dynamicdata)  [unwired: 3 in]
          n682 = call "Convert to Dynamic Data4"("Array"=w1006) -> ("Dynamic Data Type"=w1007:dynamicdata)  [unwired: 3 in]
          n683 = call "Convert to Dynamic Data2"("Array"=w998) -> ("Dynamic Data Type"=w993:dynamicdata)  [unwired: 3 in]
          n684 = Merge Signals(w992, w1007) -> (w1005:dynamicdata)
          n685 = call "Convert to Dynamic Data3"("Array"=w1003) -> ("Dynamic Data Type"=w1004:dynamicdata)  [unwired: 3 in]
          n686 = Merge Signals(w993, w1004) -> (w1002:dynamicdata)
          n687 = Merge Signals(w1005, w988) -> (w989:dynamicdata)
          n688 = Merge Signals(w1002, w987) -> (w990:dynamicdata)
          n689 = call "Build XY Graph"("Y Input"=w990, "X Input"=w989) -> ("XY Graph"=→"XY Graph":cluster{"Y":dbl[], "Y":dbl[]}[])  [unwired: 3 in, 6 out]
        }
        frame #3 {
          n690 = disable-structure shown="Disabled" {
            disable-tunnel: [w1035 _] -> w1032
            frame Disabled {
              n691 = local read "center"() -> (w1036:i16)
              n692 = disable-structure shown="Enabled" {
                disable-tunnel: [w1037 TRUE] -> w1033
                frame Disabled {
                  n693 = global read "G_VEH.vi" "candata"() -> (w1040:T4)
                  n694 = Unbundle By Name(w1040) -> ("VS_can"=w1039:dbl)
                  n695 = Greater?(x=w1039, y=5.0) -> (0:w1037:bool)
                }
                frame Enabled {
                }
              }
              n696 = Equal To 0?(x=w1036) -> (x = 0?=w1034:bool)
              n697 = And(x=w1034, y=w1033) -> ()  [unwired: 1 out]
              n698 = case shown="True" w1033 {
                tunnel: [_ w1042] -> w1035
                frame False {
                }
                frame True {
                  n699 = local read "right"() -> (w1046:i16)
                  n700 = local read "left"() -> (w1047:i16)
                  n701 = Not Equal To 0?(x=w1047) -> (x != 0?=w1045:bool)
                  n702 = Not Equal To 0?(x=w1046) -> (x != 0?=w1044:bool)
                  n703 = And(x=w1045, y=w1044) -> (x .and. y?=w1043:bool)
                  n704 = case shown="False" w1043 {
                    tunnel: [w1048 _] -> w1042
                    frame False {
                      n705 = local read "left"() -> (w1050:i16)
                      n706 = Not Equal To 0?(x=w1050) -> (x != 0?=w1049:bool)
                      n707 = case shown="True" w1049 {
                        tunnel: [w1057 w1061] -> w1048
                        frame False {
                          n708 = local read "right"() -> (w1059:i16)
                          n709 = local read "rd"() -> (w1055:dbl)
                          n710 = Not Equal To 0?(x=w1059) -> (x != 0?=w1058:bool)
                          n711 = Equal To 0?(x=w1055) -> (x = 0?=w1054:bool)
                          n712 = Select(t=-0.025, s=w1054, f=-0.075) -> (s? t:f=w1051:dbl)
                          n713 = Select(t=w1051, s=w1058, f=0.0) -> (s? t:f=w1057:dbl)
                        }
                        frame True {
                          n714 = local read "rd"() -> (w1064:dbl)
                          n715 = Equal To 0?(x=w1064) -> (x = 0?=w1063:bool)
                          n716 = Select(t=0.025, s=w1063, f=0.075) -> (s? t:f=w1061:dbl)
                        }
                      }
                    }
                    frame True {
                    }
                  }
                }
              }
            }
            frame Enabled {
            }
          }
          "shift" <- w1032
        }
      }
    }
  }
